vi "Autonomous Independent.vi"() -> ()   [LabVIEW 2016]
doc: "This VI is called when autonomous begins, and will automatically be terminated when autonomous ends. You can carry out timed or sensor driven robot movement independently without needing to return to the caller."
uses:
  <vilib>/Rock Robotics/WPI/ThirdParty/CanMotor/TalonSRX/WPI_CANTalonSRX_APIFeedbackSelect.ctl
  <vilib>/Rock Robotics/WPI/ThirdParty/CanMotor/TalonSRX/WPI_CANTalonSRX_Params.ctl
  <vilib>/Rock Robotics/WPI/ThirdParty/CanMotor/TalonSRX/WPI_CANTalonSRX_APIControlMode.ctl
  <vilib>/Rock Robotics/WPI/Utilities/WPI_GetSetVariantRefNum.vi
  <vilib>/Rock Robotics/Network Tables/NT Read String.vi
  <vilib>/Rock Robotics/Network Tables/NT Write Numeric Array.vi
  Robot Global Data.vi
  <vilib>/Rock Robotics/WPI/RobotDrive/WPI_RobotDriveArcadeDrive_Standard(NoSaturation).vi
panel:
  out "TEST 3":dbl
  out "Encoder Position 7":dbl
  out "Encoder Position 6":dbl
  out "RIGHT SIDE":dbl
  out "Encoder Position 4":dbl
  out "Encoder Position 3":dbl
  out "Encoder Position":dbl
  out "Encoder Position 2":dbl
  # "Be sure to right-click and choose Data Operations>>Make Current Value default if you want to save the array values with the VI"
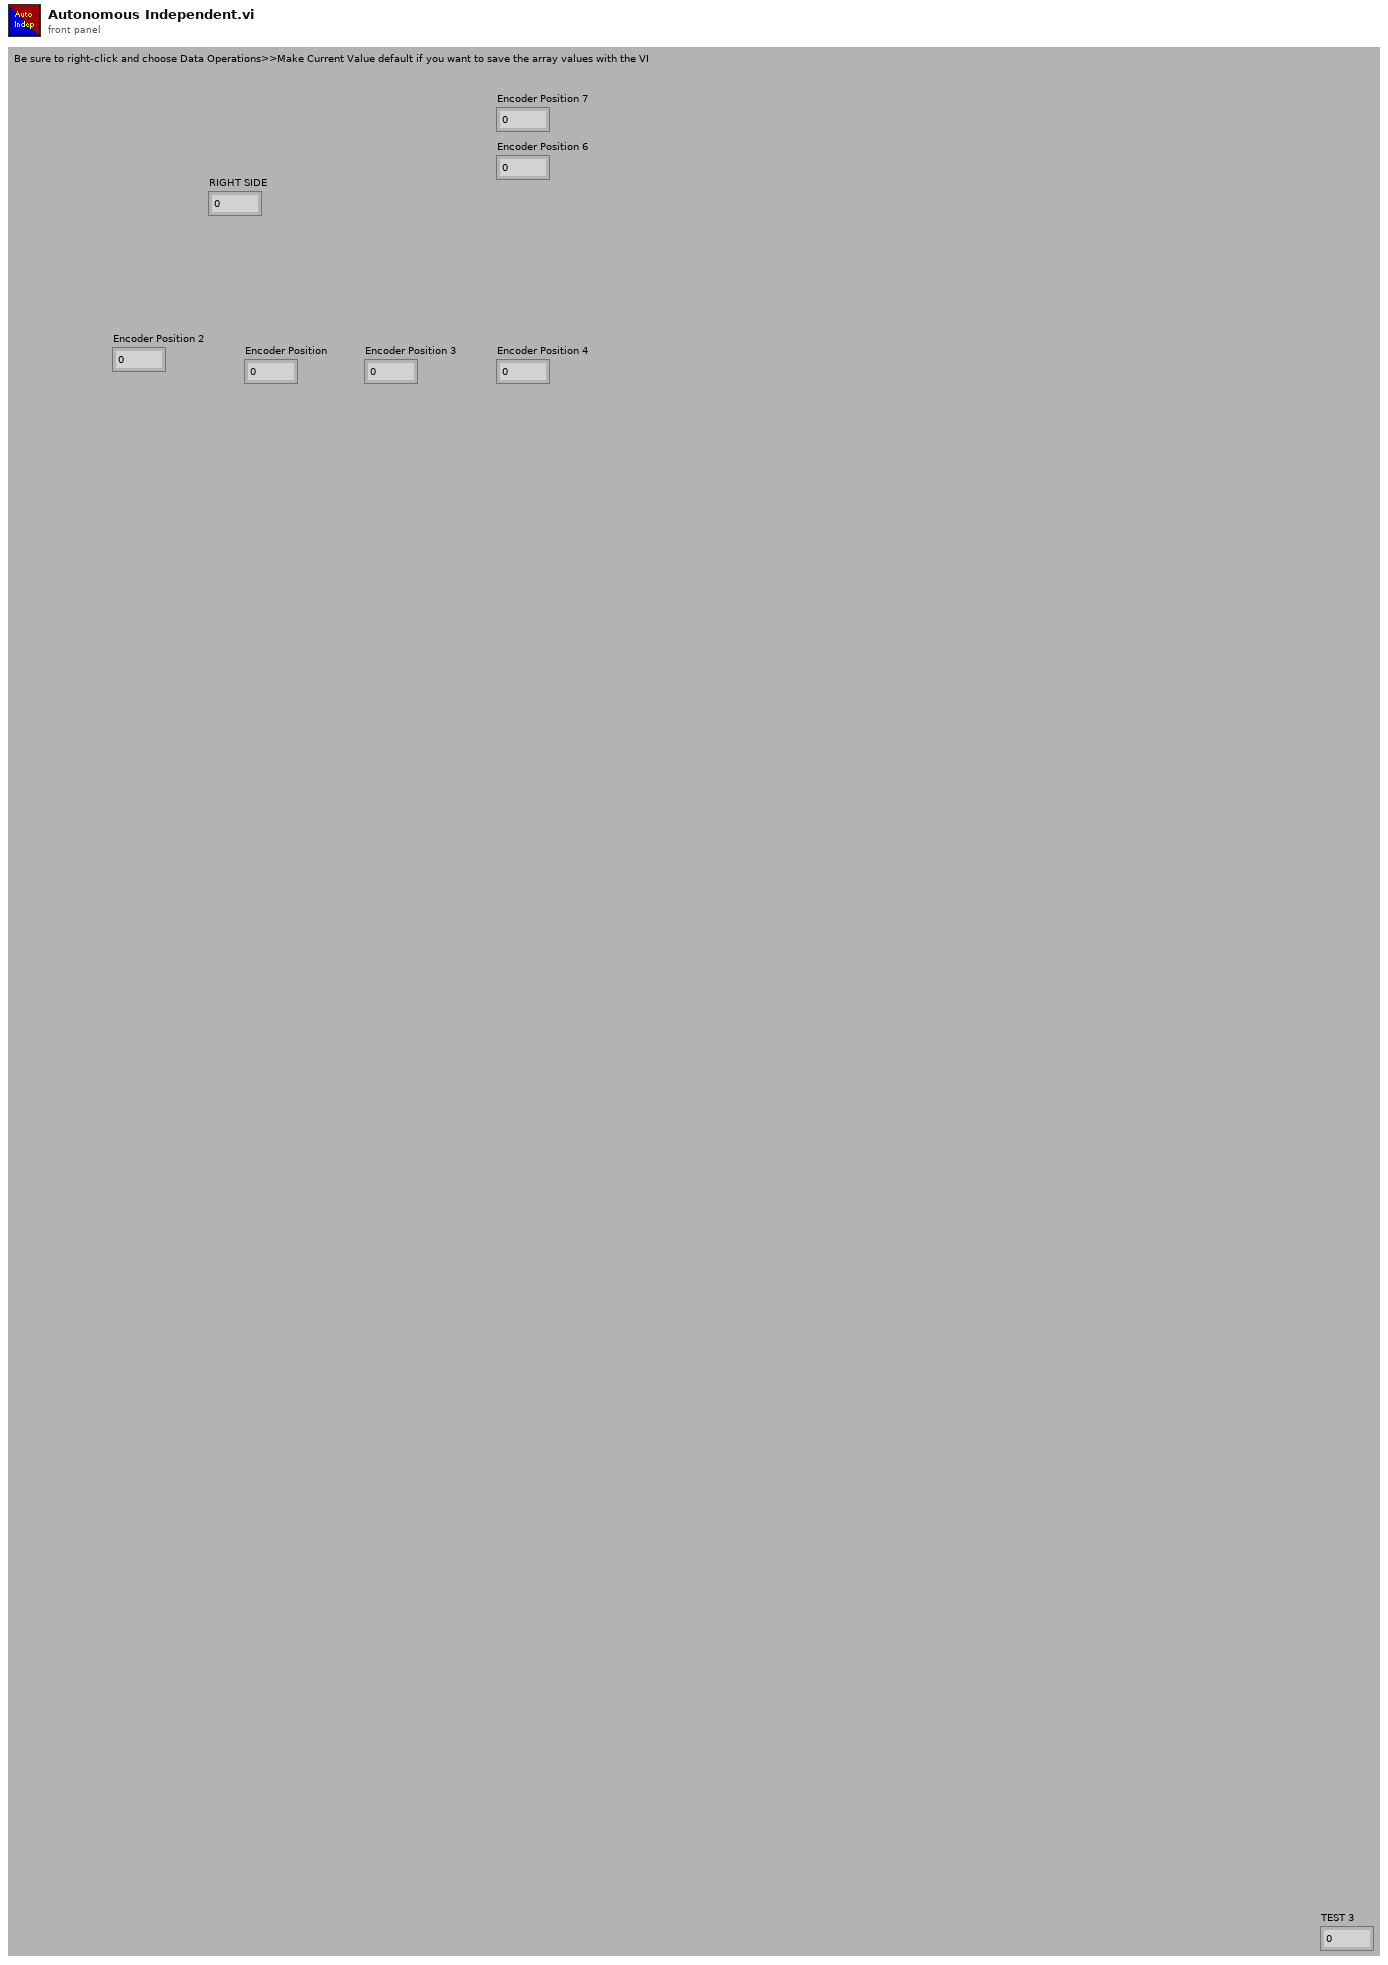
[diagram p1: front panel]
types:
  T1 = typedef "WPI_CANTalonSRX_APIFeedbackSelect.ctl" = enum16{"Digital Quadrature Encoder", "Analog Potentiometer", "Analog Encoder", "Count on Quad-A (Rising-Edge)", "Count on Quad-A (Falling-Edge)", "CTR Magnetic Enc (Absolute)", "CTR Magnetic Enc (Relative)", "Pulse Width"}
  T2 = typedef "WPI_JoystickDevRef.ctl" = cluster{"Device":T3}
  T3 = typedef "WPI_JoystickDeviceEnum.ctl" = enum16{"USB 0", "USB 1", "USB 2", "USB 3", "USB 4", "USB 5"}
  T4 = typedef "WPI_MotorControlDeviceRef.ctl" = cluster{"DeviceStatus":errorcluster, "Type":T5, "PWM":cluster{"PWM Channel":T6, "DeadBand":T7}, "CAN":cluster{"Device Number":u8, "SetOutput VI Ref":variant, "GetOutput VI Ref":variant, "Enable VI Ref":variant, "Disable VI Ref":variant, "Data":variant}, "Invert":bool}
  T5 = typedef "WPI_MotorControlType.ctl" = enum16{"PWM", "CAN"}
  T6 = typedef "FPGA_DIOPWMChannel.ctl" = enum8{"PWM 0", "PWM 1", "PWM 2", "PWM 3", "PWM 4", "PWM 5", "PWM 6", "PWM 7", "PWM 8", "PWM 9", "PWM MXP 0", "PWM MXP 1", "PWM MXP 2", "PWM MXP 3", "PWM MXP 4", "PWM MXP 5", "PWM MXP 6", "PWM MXP 7", "PWM MXP 8", "PWM MXP 9", "Invalid"}
  T7 = typedef "WPI_PWMDeadband.ctl" = cluster{"Name":string, "maxPositivePwm":i32, "minPositivePwm":i32, "centerPwm":i32, "maxNegativePwm":i32, "minNegativePwm":i32, "angularRange":u16}
  T8 = typedef "WPI_CANTalonSRX_GlobalStatus.ctl" = cluster{"Applied Throttle":dbl, "Module Enabled":bool, "CAN Error":errorcluster, "Closed Loop Error":dbl, "Forward Limit Switch Closed":bool, "Reverse Limit Switch Closed":bool, "Sensor Position":dbl, "Sensor Velocity":dbl, "Current":dbl, "Sticky Fault - Over Temp":bool, "Sticky Fault - Under Voltage":bool, "Sticky Fault - Forward Limit":bool, "Sticky Fault - Reverse Limit":bool, "Sticky Fault - Forward Soft Limit":bool, "Sticky Fault - Reverse Soft Limit":bool, "Brake is Enabled":bool, "Encoder Position":dbl, "Encoder Velocity":dbl, "Encoder Index Count":dbl, "Encoder A Pin State":bool, "Encoder B Pin State":bool, "Encoder Index Pin State":bool, "Analog In":dbl, "Analog In Velocity":dbl, "Temperature (C)":dbl, "Battery Voltage":dbl, "Control 5 Is Supported":bool, "Current Profile Slot Select":dbl, "Pos Div 8":bool, "Vel Div 4":bool, "Pulse Width Position":i32, "Pulse Width Velocity":i32, "Pulse Width Rise To Rise (us)":i32, "Pulse Width Rise To Fall (us)":i32, "Mot Prof Active Is Under Run":bool, "Mot Prof Active Has Under Run":bool, "Mot Prof Active Is Last":bool, "Mot Prof Active Velocity Only":bool, "Mot Prof Active Is Valid":bool, "Mot Prof Buffer Is Full":bool, "Mot Prof Active Profile Slot Select":i32, "Mot Prof NextID":i32, "Mot Prof Count":i32, "Mot Prof Active Velocity":dbl, "Mot Prof Active Position":dbl, "Mot Prof Output Enable":i32, "UsageFrame":u32}
  T9 = typedef "WPI_RobotDriveDevRef.ctl" = cluster{"DevStatus":errorcluster, "Motors[]":T4[], "Square Inputs":bool, "Max Output":dbl}
  T10 = typedef "WPI_CANTalonSRX_APIControlMode.ctl" = enum8{"Percent VBus", "Speed", "Position", "Slave", "Unchanged / Invalid", "Voltage Compensation", "Current", "Motion Profile", "Motion Magic"}
  T11 = typedef "WPI_CANTalonSRX_Params.ctl" = u8
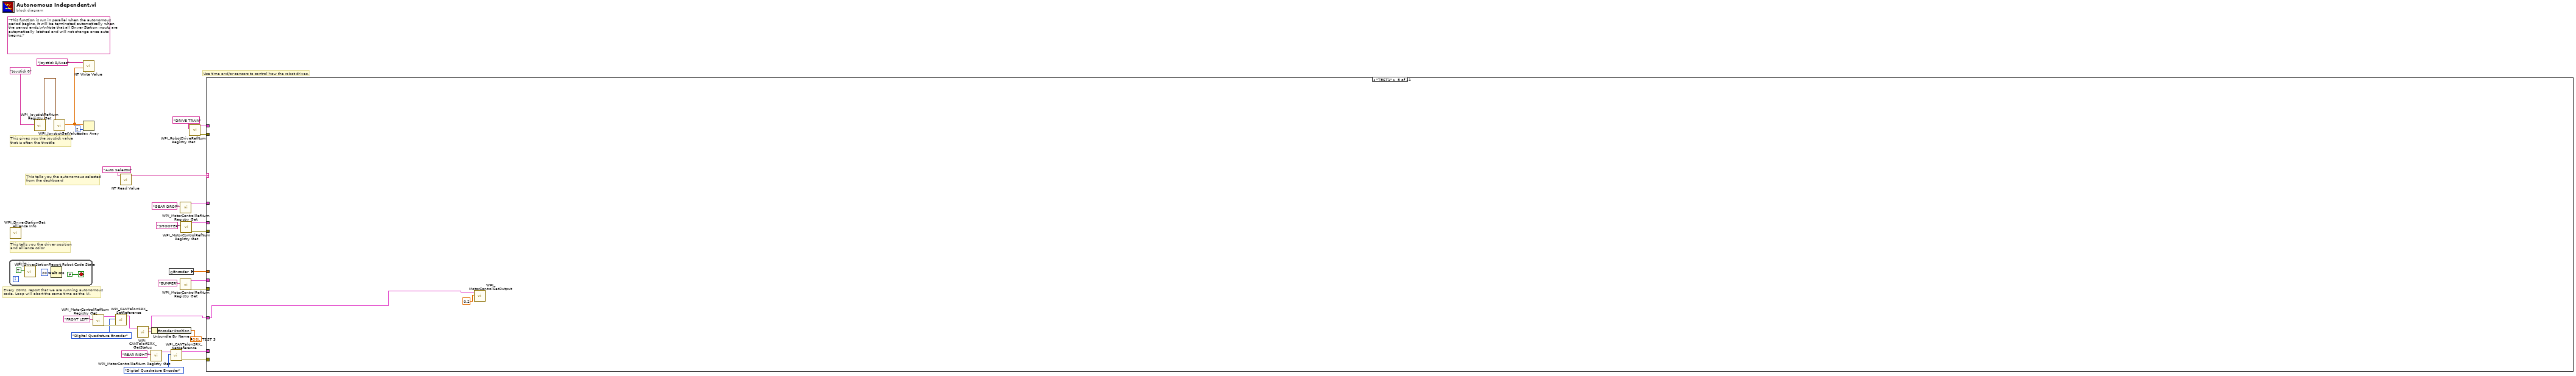
[diagram p0: block diagram]
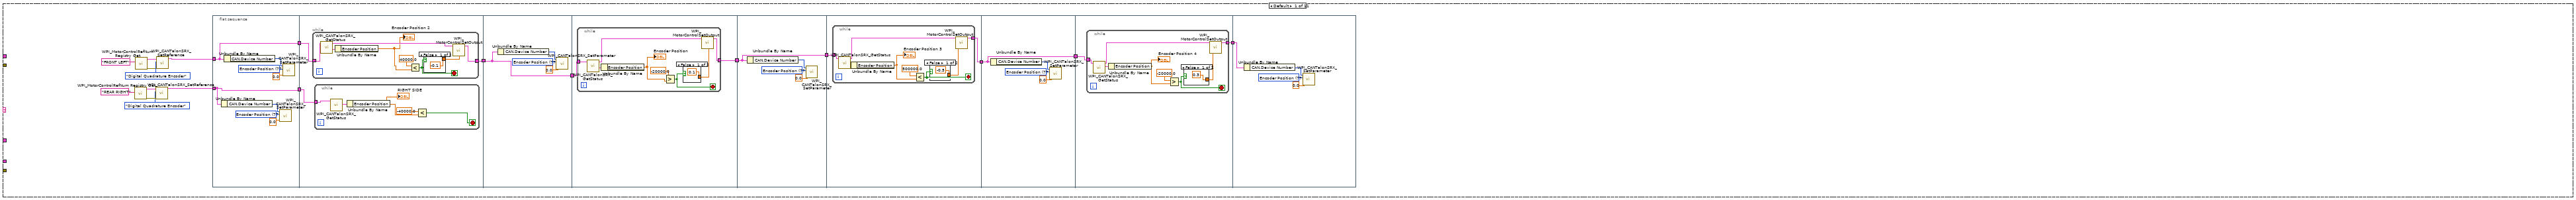
[diagram p2: hidden frame]
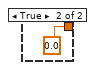
[diagram p3: hidden frame]
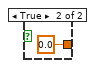
[diagram p4: hidden frame]
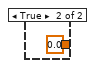
[diagram p5: hidden frame]
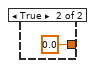
[diagram p6: hidden frame]
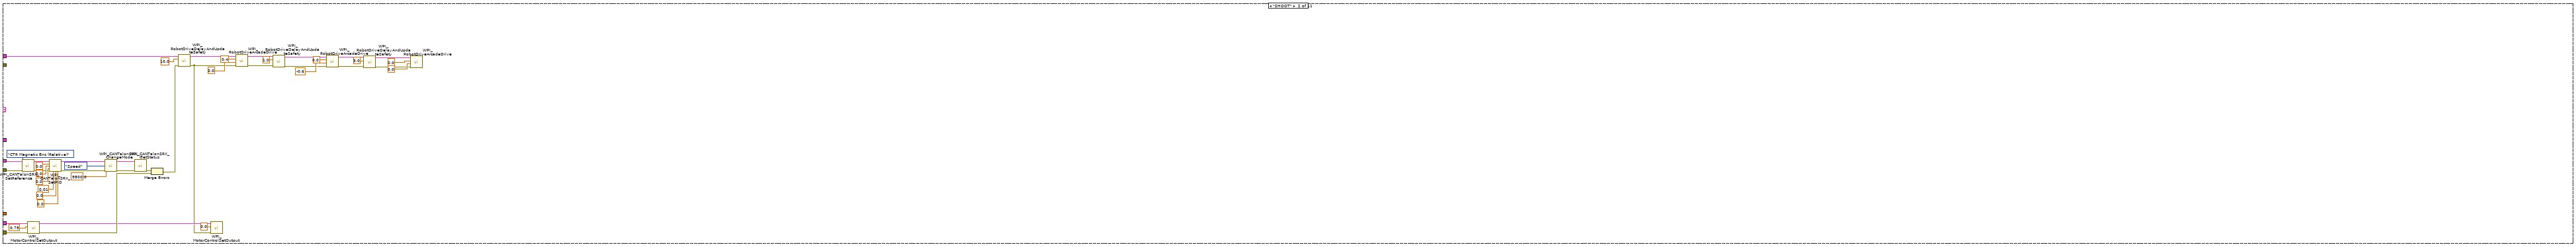
[diagram p7: hidden frame]
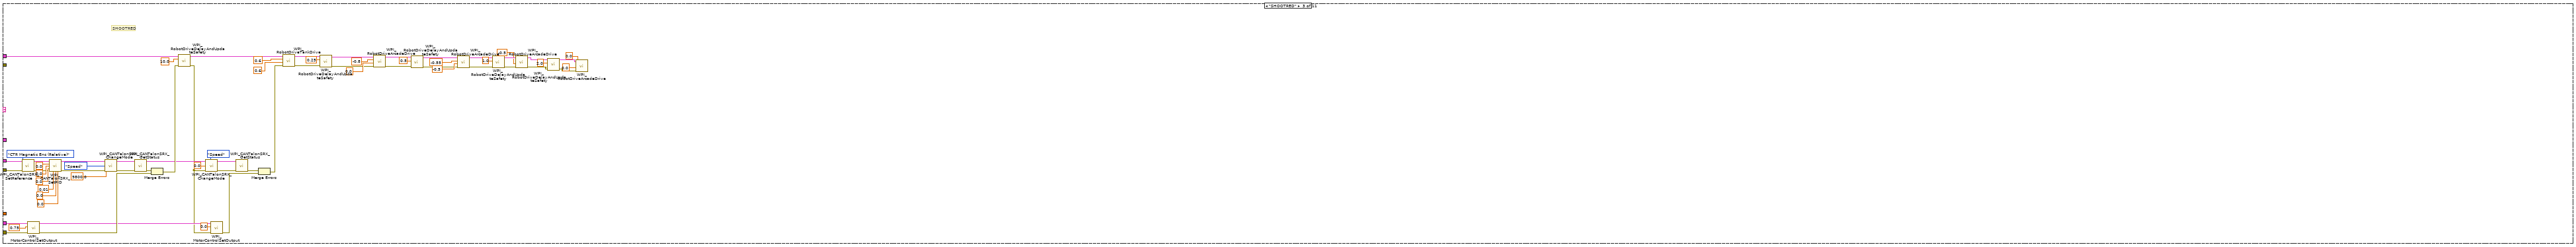
[diagram p8: hidden frame]
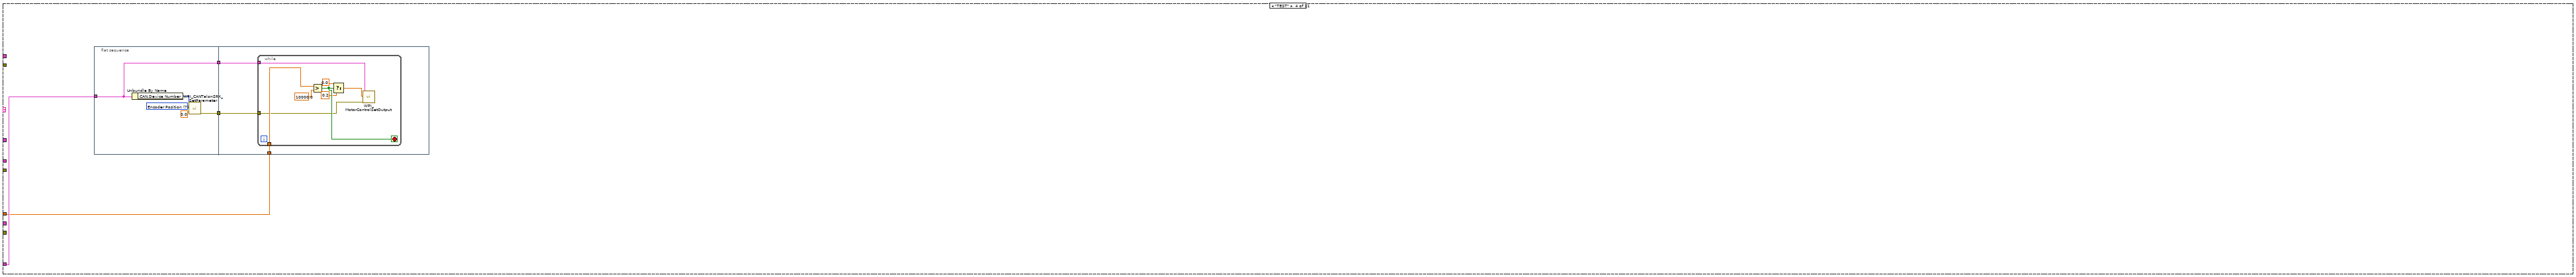
[diagram p9: hidden frame]
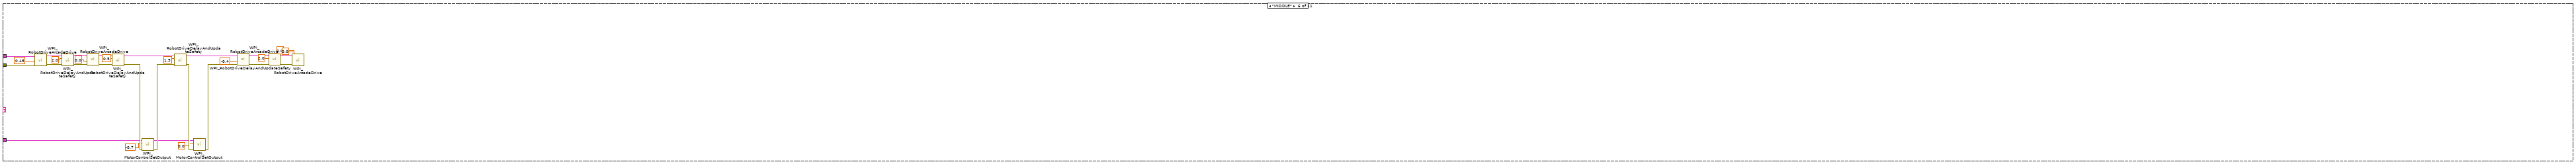
[diagram p10: hidden frame]
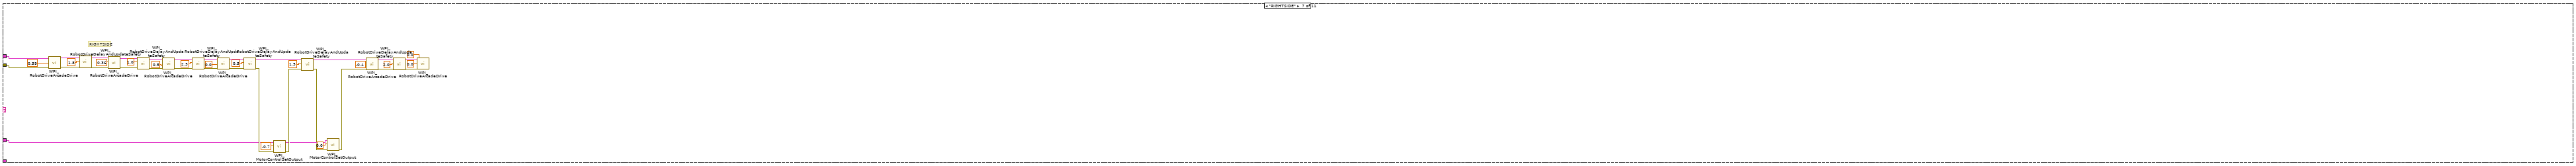
[diagram p11: hidden frame]
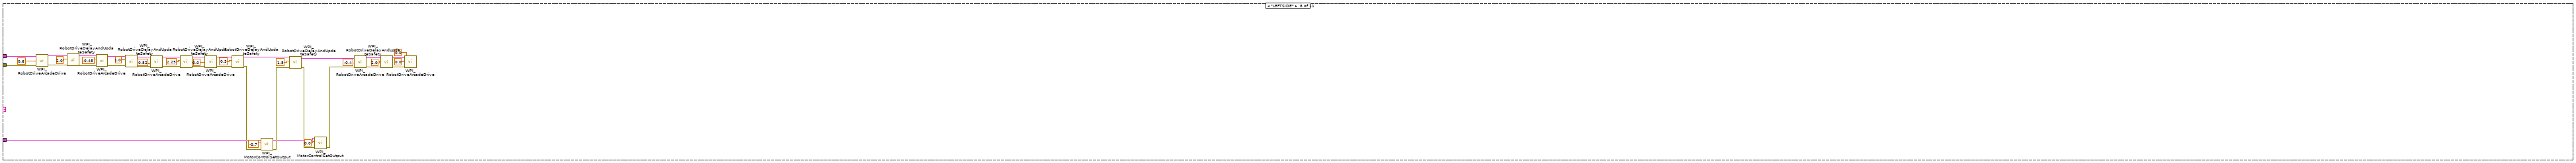
[diagram p12: hidden frame]
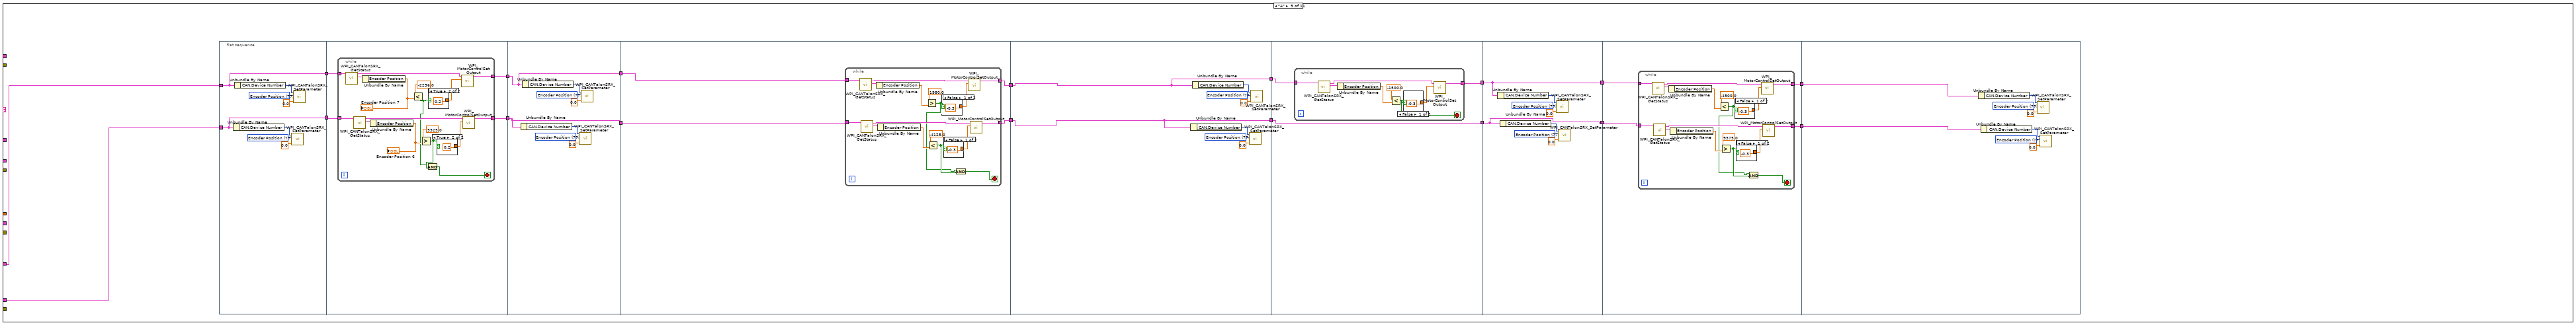
[diagram p13: hidden frame]
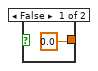
[diagram p14: hidden frame]
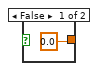
[diagram p15: hidden frame]
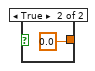
[diagram p16: hidden frame]
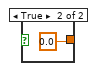
[diagram p17: hidden frame]
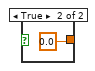
[diagram p18: hidden frame]
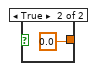
[diagram p19: hidden frame]
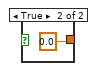
[diagram p20: hidden frame]
diagram:
  (unwired) "This function is run in parallel when the autonomous period begins. It will be terminated automatically when the period ends.\n\nNote that all Driver Station inputs are automatically latched and will not change once auto begins."
  # "Use time and/or sensors to control how the robot drives."
  # "This tells you the autonomous selected\nfrom the dashboard"
  # "Every 20ms, report that we are running autonomous\ncode. Loop will abort the same time as the VI."
  # "This gives you the joystick value\nthat is often the throttle"
  # "This tells you the driver position\nand alliance color"
  n1 = while {
    stop <- FALSE stop-if-true
    n2 = call <vilib>:"WPI_DriverStationReport Robot Code State.vi"("Autonomous"=TRUE) -> ()  [unwired: 10 in, 1 out]
    n3 = Wait (ms)(milliseconds to wait=u32 20) -> ()  [unwired: 1 out]
  }
  n4 = call <vilib>:"WPI_DriverStationGet Alliance Info.vi"() -> ()  [unwired: 12 out]
  n5 = call <vilib>:"WPI_JoystickRefNum Registry Get.vi"("refnum name"="Joystick 0") -> ("JoystickDevRef"=w31:T2)  [unwired: 1 in, 9 out]
  n6 = call <vilib>:"WPI_JoystickGetValues.vi"("JoystickDevRef"=w31) -> ("Axes"=w27:dbl[])  [unwired: 6 in, 4 out]
  n7 = call-poly <vilib>:"NT Write Value.vi"("Numeric Array"=w27, "Name"="Joystick 0/Axes") -> ()  [unwired: 9 in, 1 out]
  n8 = Index Array(array=w27, index=2) -> ()  [unwired: 1 out]
  n9 = call <vilib>:"WPI_MotorControlRefNum Registry Get.vi"("refnum name"="FRONT LEFT") -> ("error out"=w6:errorcluster, "MotorControlDevRef"=w7:T4)  [unwired: 9 in]
  n10 = call <vilib>:"WPI_CANTalonSRX_SetReference.vi"("error in (no error)"=w6, "Feedback Reference"=WPI_CANTalonSRX_APIFeedbackSelect."Digital Quadrature Encoder", "CAN Talon SRX Ref"=w7) -> ("CAN Talon SRX Ref"=w2:T4)  [unwired: 7 in, 1 out]
  n11 = call-poly <vilib>:"NT Read Value.vi"("Name"="Auto Selector") -> ("String"=w28:string)  [unwired: 9 in, 1 out]
  n12 = call <vilib>:"WPI_CANTalonSRX_GetStatus.vi"("CAN Talon SRX Ref"=w2) -> ("Talon SRX Status"=w4:T8, "CAN Talon SRX Ref"=w1:T4)  [unwired: 8 in, 1 out]
  n13 = call <vilib>:"WPI_MotorControlRefNum Registry Get.vi"("refnum name"="REAR RIGHT") -> ("MotorControlDevRef"=w23:T4)  [unwired: 9 in, 1 out]
  n14 = Unbundle By Name(w4) -> ("Encoder Position"=→"TEST 3":dbl)
  n15 = global read "Robot Global Data.vi" "Encoder"() -> (w8:dbl)
  n16 = call <vilib>:"WPI_CANTalonSRX_SetReference.vi"("Feedback Reference"=WPI_CANTalonSRX_APIFeedbackSelect."Digital Quadrature Encoder", "CAN Talon SRX Ref"=w23) -> ("error out"=w20:errorcluster, "CAN Talon SRX Ref"=w21:T4)  [unwired: 8 in]
  n17 = call <vilib>:"WPI_MotorControlRefNum Registry Get.vi"("refnum name"="GEAR DROP") -> ("MotorControlDevRef"=w15:T4)  [unwired: 9 in, 1 out]
  n18 = call <vilib>:"WPI_MotorControlRefNum Registry Get.vi"("refnum name"="BUMPER") -> ("error out"=w10:errorcluster, "MotorControlDevRef"=w11:T4)  [unwired: 9 in]
  n19 = call <vilib>:"WPI_MotorControlRefNum Registry Get.vi"("refnum name"="SHOOTER") -> ("error out"=w12:errorcluster, "MotorControlDevRef"=w13:T4)  [unwired: 9 in]
  n20 = call <vilib>:"WPI_RobotDriveRefNum Registry Get.vi"("refnum name"="DRIVE TRAIN") -> ("error out"=w17:errorcluster, "RobotDriveDevRef"=w18:T9)  [unwired: 9 in]
  n21 = case shown="\"TEST1\"" w28 {
    tunnel: w21 -> [_ _ _ _ _ _ _ _ w389 _ _]
    tunnel: w20 -> [_ _ _ _ _ _ _ _ _ _ _]
    tunnel: w18 -> [_ w159 w225 _ _ w296 w299 w382 _ w534 w559]
    tunnel: w17 -> [_ _ _ _ _ w295 w298 w381 _ w533 w558]
    tunnel: w15 -> [_ _ _ _ _ w283 w297 w358 _ _ w539]
    tunnel: w13 -> [_ w165 w231 _ _ _ _ _ _ _ _]
    tunnel: w12 -> [_ w164 w230 _ _ _ _ _ _ _ _]
    tunnel: w11 -> [_ w150 w218 _ _ _ _ _ _ _ _]
    tunnel: w10 -> [_ w149 w217 _ _ _ _ _ _ _ _]
    tunnel: w1 -> [_ _ _ w247 w264 _ _ _ w384 _ _]
    tunnel: w8 -> [_ _ _ w246 _ _ _ _ _ _ _]
    frame Default {
      n22 = call <vilib>:"WPI_MotorControlRefNum Registry Get.vi"("refnum name"="REAR RIGHT") -> ("error out"=w40:errorcluster, "MotorControlDevRef"=w39:T4)  [unwired: 9 in]
      n23 = call <vilib>:"WPI_MotorControlRefNum Registry Get.vi"("refnum name"="FRONT LEFT") -> ("error out"=w52:errorcluster, "MotorControlDevRef"=w53:T4)  [unwired: 9 in]
      n24 = call <vilib>:"WPI_CANTalonSRX_SetReference.vi"("error in (no error)"=w40, "Feedback Reference"=WPI_CANTalonSRX_APIFeedbackSelect."Digital Quadrature Encoder", "CAN Talon SRX Ref"=w39) -> ("CAN Talon SRX Ref"=w37:T4)  [unwired: 7 in, 1 out]
      n25 = call <vilib>:"WPI_CANTalonSRX_SetReference.vi"("error in (no error)"=w52, "Feedback Reference"=WPI_CANTalonSRX_APIFeedbackSelect."Digital Quadrature Encoder", "CAN Talon SRX Ref"=w53) -> ("CAN Talon SRX Ref"=w48:T4)  [unwired: 7 in, 1 out]
      n26 = flat-sequence {
        tunnel: w48 -> [w59]
        tunnel: [w59] -> w47
        tunnel: w37 -> [w55]
        tunnel: [w55] -> w36
        tunnel: [w64] -> w50
        tunnel: w47 -> [w65]
        tunnel: w36 -> [w63]
        tunnel: w50 -> [w81]
        tunnel: [w81] -> w49
        tunnel: w49 -> [w86]
        tunnel: [w85] -> w46
        tunnel: w46 -> [w97]
        tunnel: [w97] -> w45
        tunnel: w45 -> [w102]
        tunnel: [w101] -> w44
        tunnel: w44 -> [w113]
        tunnel: [w113] -> w43
        tunnel: w43 -> [w118]
        tunnel: [w117] -> w42
        tunnel: w42 -> [w129]
        frame #0 {
          w57 = T11 77 items=["Slot 0 - P"=1, "Slot 0 - I"=2, "Slot 0 - D"=3, "Slot 0 - F"=4, "Slot 0 - I Zone"=5, "Slot 0 - Ramp Rate"=6, "Slot 1 - P"=11, "Slot 1 - I"=12, "Slot 1 - D"=13, "Slot 1 - F"=14, "Slot 1 - I Zone"=15, "Slot 1 - Ramp Rate"=16, "Soft Limit - Forward"=21, "Soft Limit - Reverse"=22, "Soft Limit - Forward Enable"=23, "Soft Limit - Reverse Enable"=24, "On Boot - Brake Mode"=31, "On Boot - Limit Normally Closed - Forward"=32, "On Boot - Limit Normally Closed - Reverse"=33, "On Boot - Limit Disabled - Forward"=34, "On Boot - Limit Disabled - Reverse"=35, "Fault - Over Temp"=41, "Fault - Under Voltage"=42, "Fault - Forward Limit"=43, "Fault - Reverse Limit"=44, "Fault - Hardware Failure"=45, "Fault - Forward Soft Limit"=46, "Fault - Reverse Soft Limit"=47, "Sticky Fault - Over Temp"=48, "Sticky Fault - Under Voltage"=49, "Sticky Fault - Forward Limit"=50, "Sticky Fault - Reverse Limit"=51, "Sticky Fault - Forward Soft Limit"=52, "Sticky Fault - Reverse Soft Limit"=53, "Applied Throttle"=61, "Closed-Loop Error"=62, "Select Feedback Device"=63, "Reverse Closed-Loop Output"=64, "Mode Select"=65, "Profile Slot Select"=66, "Ramp Throttle"=67, "Reverse Feedback Sensor"=68, "Limit Switch Enabled"=69, "Limit Switch Closed - Forward"=70, "Limit Switch Closed - Reverse"=71, "Sensor Position"=73, "Sensor Velocity"=74, "Current"=75, "Brake is Enabled"=76, "Encoder Position"=77, "Encoder Velocity"=78, "Encoder Index Rise Events"=79, "Encoder A Pin State"=80, "Encoder B Pin State"=81, "Encoder Index Pin State"=82, "Analog In with Overflow"=83, "Analog In Velocity"=84, "Temperature"=85, "Battery Voltage"=86, "Reset Count"=87, "Reset Flags"=88, "Firmware Version"=89, "Settings Changed"=90, "Quad Filter Enable"=91, "Ignore Disable Broadcast"=92, "I Accumulator"=93, "Status 1 Frame Rate Ms"=94, "Status 2 Frame Rate Ms"=95, "Status 3 Frame Rate Ms"=96, "Status 4 Frame Rate Ms"=97, "Status 6 Frame Rate Ms"=98, "Status 7 Frame Rate Ms"=99, "Enable Index Pin Clear Position"=100, "Peak Positive Output"=104, "Nominal Positive Output"=105, "Peak Negative Output"=106, "Nominal Negative Output"=107, "Quad Index Pin Polarity"=108, "Status 8 Frame Rate Ms"=109, "Allow Position Overflow"=110, "Slot 0 - Allowable Closed-Loop Error"=111, "Number Potentiometer Turns"=112, "Encoder Codes Per Rev"=113, "Pulse Width Decoded Position"=114, "Analog Position"=115, "Voltage Compensation Rate (V/s)"=116, "Slot 1 - Allowable Closed-Loop Error"=117, "Motion Profile Has Underrun Err"=119, "Reserved 120"=120, "Legacy Control Mode"=121, "Motion Magic Acceleration"=122, "Motion Magic Cruise Velocity"=123, "Status 10 Frame Rate"=124, "Current Limit Threshold"=125, "CustomParam0"=137, "CustomParam1"=138, "PersStorageSaving"=139, "ClearPositionOnLimitF"=144, "ClearPositionOnLimitR"=145, "NominalBatteryVoltage"=146, "SampleVelocityPeriod"=147, "SampleVelocityWindow"=148] ("Parameter")
          w61 = T11 77 items=["Slot 0 - P"=1, "Slot 0 - I"=2, "Slot 0 - D"=3, "Slot 0 - F"=4, "Slot 0 - I Zone"=5, "Slot 0 - Ramp Rate"=6, "Slot 1 - P"=11, "Slot 1 - I"=12, "Slot 1 - D"=13, "Slot 1 - F"=14, "Slot 1 - I Zone"=15, "Slot 1 - Ramp Rate"=16, "Soft Limit - Forward"=21, "Soft Limit - Reverse"=22, "Soft Limit - Forward Enable"=23, "Soft Limit - Reverse Enable"=24, "On Boot - Brake Mode"=31, "On Boot - Limit Normally Closed - Forward"=32, "On Boot - Limit Normally Closed - Reverse"=33, "On Boot - Limit Disabled - Forward"=34, "On Boot - Limit Disabled - Reverse"=35, "Fault - Over Temp"=41, "Fault - Under Voltage"=42, "Fault - Forward Limit"=43, "Fault - Reverse Limit"=44, "Fault - Hardware Failure"=45, "Fault - Forward Soft Limit"=46, "Fault - Reverse Soft Limit"=47, "Sticky Fault - Over Temp"=48, "Sticky Fault - Under Voltage"=49, "Sticky Fault - Forward Limit"=50, "Sticky Fault - Reverse Limit"=51, "Sticky Fault - Forward Soft Limit"=52, "Sticky Fault - Reverse Soft Limit"=53, "Applied Throttle"=61, "Closed-Loop Error"=62, "Select Feedback Device"=63, "Reverse Closed-Loop Output"=64, "Mode Select"=65, "Profile Slot Select"=66, "Ramp Throttle"=67, "Reverse Feedback Sensor"=68, "Limit Switch Enabled"=69, "Limit Switch Closed - Forward"=70, "Limit Switch Closed - Reverse"=71, "Sensor Position"=73, "Sensor Velocity"=74, "Current"=75, "Brake is Enabled"=76, "Encoder Position"=77, "Encoder Velocity"=78, "Encoder Index Rise Events"=79, "Encoder A Pin State"=80, "Encoder B Pin State"=81, "Encoder Index Pin State"=82, "Analog In with Overflow"=83, "Analog In Velocity"=84, "Temperature"=85, "Battery Voltage"=86, "Reset Count"=87, "Reset Flags"=88, "Firmware Version"=89, "Settings Changed"=90, "Quad Filter Enable"=91, "Ignore Disable Broadcast"=92, "I Accumulator"=93, "Status 1 Frame Rate Ms"=94, "Status 2 Frame Rate Ms"=95, "Status 3 Frame Rate Ms"=96, "Status 4 Frame Rate Ms"=97, "Status 6 Frame Rate Ms"=98, "Status 7 Frame Rate Ms"=99, "Enable Index Pin Clear Position"=100, "Peak Positive Output"=104, "Nominal Positive Output"=105, "Peak Negative Output"=106, "Nominal Negative Output"=107, "Quad Index Pin Polarity"=108, "Status 8 Frame Rate Ms"=109, "Allow Position Overflow"=110, "Slot 0 - Allowable Closed-Loop Error"=111, "Number Potentiometer Turns"=112, "Encoder Codes Per Rev"=113, "Pulse Width Decoded Position"=114, "Analog Position"=115, "Voltage Compensation Rate (V/s)"=116, "Slot 1 - Allowable Closed-Loop Error"=117, "Motion Profile Has Underrun Err"=119, "Reserved 120"=120, "Legacy Control Mode"=121, "Motion Magic Acceleration"=122, "Motion Magic Cruise Velocity"=123, "Status 10 Frame Rate"=124, "Current Limit Threshold"=125, "CustomParam0"=137, "CustomParam1"=138, "PersStorageSaving"=139, "ClearPositionOnLimitF"=144, "ClearPositionOnLimitR"=145, "NominalBatteryVoltage"=146, "SampleVelocityPeriod"=147, "SampleVelocityWindow"=148] ("Parameter")
          n27 = Unbundle By Name(w55) -> ("CAN.Device Number"=w56:u8)
          n28 = Unbundle By Name(w59) -> ("CAN.Device Number"=w62:u8)
          n29 = call <vilib>:"WPI_CANTalonSRX_SetParameter.vi"("Value"=0.0, "Parameter"=w57, "Device ID (0)"=w56) -> ()  [unwired: 7 in, 2 out]
          n30 = call <vilib>:"WPI_CANTalonSRX_SetParameter.vi"("Value"=0.0, "Parameter"=w61, "Device ID (0)"=w62) -> ()  [unwired: 7 in, 2 out]
        }
        frame #1 {
          n31 = while {
            tunnel: w65 -> [w72]
            tunnel: [w71] -> w64
            stop <- w75 stop-if-true
            n32 = call <vilib>:"WPI_CANTalonSRX_GetStatus.vi"("CAN Talon SRX Ref"=w72) -> ("Talon SRX Status"=w78:T8, "CAN Talon SRX Ref"=w77:T4)  [unwired: 8 in, 1 out]
            n33 = Unbundle By Name(w78) -> ("Encoder Position"=w74:dbl)
            "Encoder Position 2" <- w74
            n34 = Less?(x=40000.0, y=w74) -> (x < y?=w75:bool)
            n35 = case shown="False" w75 {
              tunnel: [-0.1 ("x") 0.0 ("x")] -> w76
              frame False {
              }
              frame True {
              }
            }
            n36 = call <vilib>:"WPI_MotorControlSetOutput.vi"("Output"=w76, "MotorControlDevRef"=w77) -> ("MotorControlDevRef"=w71:T4)  [unwired: 7 in, 2 out]
          }
          n37 = while {
            tunnel: w63 -> [w70]
            stop <- w67 stop-if-true
            n38 = call <vilib>:"WPI_CANTalonSRX_GetStatus.vi"("CAN Talon SRX Ref"=w70) -> ("Talon SRX Status"=w66:T8)  [unwired: 8 in, 2 out]
            n39 = Unbundle By Name(w66) -> ("Encoder Position"=w69:dbl)
            "RIGHT SIDE" <- w69
            n40 = Less?(x=-40000.0, y=w69) -> (x < y?=w67:bool)
          }
        }
        frame #2 {
          w83 = T11 77 items=["Slot 0 - P"=1, "Slot 0 - I"=2, "Slot 0 - D"=3, "Slot 0 - F"=4, "Slot 0 - I Zone"=5, "Slot 0 - Ramp Rate"=6, "Slot 1 - P"=11, "Slot 1 - I"=12, "Slot 1 - D"=13, "Slot 1 - F"=14, "Slot 1 - I Zone"=15, "Slot 1 - Ramp Rate"=16, "Soft Limit - Forward"=21, "Soft Limit - Reverse"=22, "Soft Limit - Forward Enable"=23, "Soft Limit - Reverse Enable"=24, "On Boot - Brake Mode"=31, "On Boot - Limit Normally Closed - Forward"=32, "On Boot - Limit Normally Closed - Reverse"=33, "On Boot - Limit Disabled - Forward"=34, "On Boot - Limit Disabled - Reverse"=35, "Fault - Over Temp"=41, "Fault - Under Voltage"=42, "Fault - Forward Limit"=43, "Fault - Reverse Limit"=44, "Fault - Hardware Failure"=45, "Fault - Forward Soft Limit"=46, "Fault - Reverse Soft Limit"=47, "Sticky Fault - Over Temp"=48, "Sticky Fault - Under Voltage"=49, "Sticky Fault - Forward Limit"=50, "Sticky Fault - Reverse Limit"=51, "Sticky Fault - Forward Soft Limit"=52, "Sticky Fault - Reverse Soft Limit"=53, "Applied Throttle"=61, "Closed-Loop Error"=62, "Select Feedback Device"=63, "Reverse Closed-Loop Output"=64, "Mode Select"=65, "Profile Slot Select"=66, "Ramp Throttle"=67, "Reverse Feedback Sensor"=68, "Limit Switch Enabled"=69, "Limit Switch Closed - Forward"=70, "Limit Switch Closed - Reverse"=71, "Sensor Position"=73, "Sensor Velocity"=74, "Current"=75, "Brake is Enabled"=76, "Encoder Position"=77, "Encoder Velocity"=78, "Encoder Index Rise Events"=79, "Encoder A Pin State"=80, "Encoder B Pin State"=81, "Encoder Index Pin State"=82, "Analog In with Overflow"=83, "Analog In Velocity"=84, "Temperature"=85, "Battery Voltage"=86, "Reset Count"=87, "Reset Flags"=88, "Firmware Version"=89, "Settings Changed"=90, "Quad Filter Enable"=91, "Ignore Disable Broadcast"=92, "I Accumulator"=93, "Status 1 Frame Rate Ms"=94, "Status 2 Frame Rate Ms"=95, "Status 3 Frame Rate Ms"=96, "Status 4 Frame Rate Ms"=97, "Status 6 Frame Rate Ms"=98, "Status 7 Frame Rate Ms"=99, "Enable Index Pin Clear Position"=100, "Peak Positive Output"=104, "Nominal Positive Output"=105, "Peak Negative Output"=106, "Nominal Negative Output"=107, "Quad Index Pin Polarity"=108, "Status 8 Frame Rate Ms"=109, "Allow Position Overflow"=110, "Slot 0 - Allowable Closed-Loop Error"=111, "Number Potentiometer Turns"=112, "Encoder Codes Per Rev"=113, "Pulse Width Decoded Position"=114, "Analog Position"=115, "Voltage Compensation Rate (V/s)"=116, "Slot 1 - Allowable Closed-Loop Error"=117, "Motion Profile Has Underrun Err"=119, "Reserved 120"=120, "Legacy Control Mode"=121, "Motion Magic Acceleration"=122, "Motion Magic Cruise Velocity"=123, "Status 10 Frame Rate"=124, "Current Limit Threshold"=125, "CustomParam0"=137, "CustomParam1"=138, "PersStorageSaving"=139, "ClearPositionOnLimitF"=144, "ClearPositionOnLimitR"=145, "NominalBatteryVoltage"=146, "SampleVelocityPeriod"=147, "SampleVelocityWindow"=148] ("Parameter")
          n41 = Unbundle By Name(w81) -> ("CAN.Device Number"=w84:u8)
          n42 = call <vilib>:"WPI_CANTalonSRX_SetParameter.vi"("Value"=0.0, "Parameter"=w83, "Device ID (0)"=w84) -> ()  [unwired: 7 in, 2 out]
        }
        frame #3 {
          n43 = while {
            tunnel: w86 -> [w88]
            tunnel: [w87] -> w85
            stop <- w91 stop-if-true
            n44 = call <vilib>:"WPI_CANTalonSRX_GetStatus.vi"("CAN Talon SRX Ref"=w88) -> ("Talon SRX Status"=w94:T8, "CAN Talon SRX Ref"=w93:T4)  [unwired: 8 in, 1 out]
            n45 = Unbundle By Name(w94) -> ("Encoder Position"=w90:dbl)
            "Encoder Position" <- w90
            n46 = Greater?(x=-20000.0 ("y"), y=w90) -> (0:w91:bool)
            n47 = case shown="False" w91 {
              tunnel: [0.1 ("x") 0.0 ("x")] -> w92
              frame False {
              }
              frame True {
              }
            }
            n48 = call <vilib>:"WPI_MotorControlSetOutput.vi"("Output"=w92, "MotorControlDevRef"=w93) -> ("MotorControlDevRef"=w87:T4)  [unwired: 7 in, 2 out]
          }
        }
        frame #4 {
          w99 = T11 77 items=["Slot 0 - P"=1, "Slot 0 - I"=2, "Slot 0 - D"=3, "Slot 0 - F"=4, "Slot 0 - I Zone"=5, "Slot 0 - Ramp Rate"=6, "Slot 1 - P"=11, "Slot 1 - I"=12, "Slot 1 - D"=13, "Slot 1 - F"=14, "Slot 1 - I Zone"=15, "Slot 1 - Ramp Rate"=16, "Soft Limit - Forward"=21, "Soft Limit - Reverse"=22, "Soft Limit - Forward Enable"=23, "Soft Limit - Reverse Enable"=24, "On Boot - Brake Mode"=31, "On Boot - Limit Normally Closed - Forward"=32, "On Boot - Limit Normally Closed - Reverse"=33, "On Boot - Limit Disabled - Forward"=34, "On Boot - Limit Disabled - Reverse"=35, "Fault - Over Temp"=41, "Fault - Under Voltage"=42, "Fault - Forward Limit"=43, "Fault - Reverse Limit"=44, "Fault - Hardware Failure"=45, "Fault - Forward Soft Limit"=46, "Fault - Reverse Soft Limit"=47, "Sticky Fault - Over Temp"=48, "Sticky Fault - Under Voltage"=49, "Sticky Fault - Forward Limit"=50, "Sticky Fault - Reverse Limit"=51, "Sticky Fault - Forward Soft Limit"=52, "Sticky Fault - Reverse Soft Limit"=53, "Applied Throttle"=61, "Closed-Loop Error"=62, "Select Feedback Device"=63, "Reverse Closed-Loop Output"=64, "Mode Select"=65, "Profile Slot Select"=66, "Ramp Throttle"=67, "Reverse Feedback Sensor"=68, "Limit Switch Enabled"=69, "Limit Switch Closed - Forward"=70, "Limit Switch Closed - Reverse"=71, "Sensor Position"=73, "Sensor Velocity"=74, "Current"=75, "Brake is Enabled"=76, "Encoder Position"=77, "Encoder Velocity"=78, "Encoder Index Rise Events"=79, "Encoder A Pin State"=80, "Encoder B Pin State"=81, "Encoder Index Pin State"=82, "Analog In with Overflow"=83, "Analog In Velocity"=84, "Temperature"=85, "Battery Voltage"=86, "Reset Count"=87, "Reset Flags"=88, "Firmware Version"=89, "Settings Changed"=90, "Quad Filter Enable"=91, "Ignore Disable Broadcast"=92, "I Accumulator"=93, "Status 1 Frame Rate Ms"=94, "Status 2 Frame Rate Ms"=95, "Status 3 Frame Rate Ms"=96, "Status 4 Frame Rate Ms"=97, "Status 6 Frame Rate Ms"=98, "Status 7 Frame Rate Ms"=99, "Enable Index Pin Clear Position"=100, "Peak Positive Output"=104, "Nominal Positive Output"=105, "Peak Negative Output"=106, "Nominal Negative Output"=107, "Quad Index Pin Polarity"=108, "Status 8 Frame Rate Ms"=109, "Allow Position Overflow"=110, "Slot 0 - Allowable Closed-Loop Error"=111, "Number Potentiometer Turns"=112, "Encoder Codes Per Rev"=113, "Pulse Width Decoded Position"=114, "Analog Position"=115, "Voltage Compensation Rate (V/s)"=116, "Slot 1 - Allowable Closed-Loop Error"=117, "Motion Profile Has Underrun Err"=119, "Reserved 120"=120, "Legacy Control Mode"=121, "Motion Magic Acceleration"=122, "Motion Magic Cruise Velocity"=123, "Status 10 Frame Rate"=124, "Current Limit Threshold"=125, "CustomParam0"=137, "CustomParam1"=138, "PersStorageSaving"=139, "ClearPositionOnLimitF"=144, "ClearPositionOnLimitR"=145, "NominalBatteryVoltage"=146, "SampleVelocityPeriod"=147, "SampleVelocityWindow"=148] ("Parameter")
          n49 = Unbundle By Name(w97) -> ("CAN.Device Number"=w100:u8)
          n50 = call <vilib>:"WPI_CANTalonSRX_SetParameter.vi"("Value"=0.0, "Parameter"=w99, "Device ID (0)"=w100) -> ()  [unwired: 7 in, 2 out]
        }
        frame #5 {
          n51 = while {
            tunnel: w102 -> [w104]
            tunnel: [w103] -> w101
            stop <- w107 stop-if-true
            n52 = call <vilib>:"WPI_CANTalonSRX_GetStatus.vi"("CAN Talon SRX Ref"=w104) -> ("Talon SRX Status"=w110:T8, "CAN Talon SRX Ref"=w109:T4)  [unwired: 8 in, 1 out]
            n53 = Unbundle By Name(w110) -> ("Encoder Position"=w106:dbl)
            "Encoder Position 3" <- w106
            n54 = Less?(x=500000.0, y=w106) -> (x < y?=w107:bool)
            n55 = case shown="False" w107 {
              tunnel: [-0.5 ("x") 0.0 ("x")] -> w108
              frame False {
              }
              frame True {
              }
            }
            n56 = call <vilib>:"WPI_MotorControlSetOutput.vi"("Output"=w108, "MotorControlDevRef"=w109) -> ("MotorControlDevRef"=w103:T4)  [unwired: 7 in, 2 out]
          }
        }
        frame #6 {
          w115 = T11 77 items=["Slot 0 - P"=1, "Slot 0 - I"=2, "Slot 0 - D"=3, "Slot 0 - F"=4, "Slot 0 - I Zone"=5, "Slot 0 - Ramp Rate"=6, "Slot 1 - P"=11, "Slot 1 - I"=12, "Slot 1 - D"=13, "Slot 1 - F"=14, "Slot 1 - I Zone"=15, "Slot 1 - Ramp Rate"=16, "Soft Limit - Forward"=21, "Soft Limit - Reverse"=22, "Soft Limit - Forward Enable"=23, "Soft Limit - Reverse Enable"=24, "On Boot - Brake Mode"=31, "On Boot - Limit Normally Closed - Forward"=32, "On Boot - Limit Normally Closed - Reverse"=33, "On Boot - Limit Disabled - Forward"=34, "On Boot - Limit Disabled - Reverse"=35, "Fault - Over Temp"=41, "Fault - Under Voltage"=42, "Fault - Forward Limit"=43, "Fault - Reverse Limit"=44, "Fault - Hardware Failure"=45, "Fault - Forward Soft Limit"=46, "Fault - Reverse Soft Limit"=47, "Sticky Fault - Over Temp"=48, "Sticky Fault - Under Voltage"=49, "Sticky Fault - Forward Limit"=50, "Sticky Fault - Reverse Limit"=51, "Sticky Fault - Forward Soft Limit"=52, "Sticky Fault - Reverse Soft Limit"=53, "Applied Throttle"=61, "Closed-Loop Error"=62, "Select Feedback Device"=63, "Reverse Closed-Loop Output"=64, "Mode Select"=65, "Profile Slot Select"=66, "Ramp Throttle"=67, "Reverse Feedback Sensor"=68, "Limit Switch Enabled"=69, "Limit Switch Closed - Forward"=70, "Limit Switch Closed - Reverse"=71, "Sensor Position"=73, "Sensor Velocity"=74, "Current"=75, "Brake is Enabled"=76, "Encoder Position"=77, "Encoder Velocity"=78, "Encoder Index Rise Events"=79, "Encoder A Pin State"=80, "Encoder B Pin State"=81, "Encoder Index Pin State"=82, "Analog In with Overflow"=83, "Analog In Velocity"=84, "Temperature"=85, "Battery Voltage"=86, "Reset Count"=87, "Reset Flags"=88, "Firmware Version"=89, "Settings Changed"=90, "Quad Filter Enable"=91, "Ignore Disable Broadcast"=92, "I Accumulator"=93, "Status 1 Frame Rate Ms"=94, "Status 2 Frame Rate Ms"=95, "Status 3 Frame Rate Ms"=96, "Status 4 Frame Rate Ms"=97, "Status 6 Frame Rate Ms"=98, "Status 7 Frame Rate Ms"=99, "Enable Index Pin Clear Position"=100, "Peak Positive Output"=104, "Nominal Positive Output"=105, "Peak Negative Output"=106, "Nominal Negative Output"=107, "Quad Index Pin Polarity"=108, "Status 8 Frame Rate Ms"=109, "Allow Position Overflow"=110, "Slot 0 - Allowable Closed-Loop Error"=111, "Number Potentiometer Turns"=112, "Encoder Codes Per Rev"=113, "Pulse Width Decoded Position"=114, "Analog Position"=115, "Voltage Compensation Rate (V/s)"=116, "Slot 1 - Allowable Closed-Loop Error"=117, "Motion Profile Has Underrun Err"=119, "Reserved 120"=120, "Legacy Control Mode"=121, "Motion Magic Acceleration"=122, "Motion Magic Cruise Velocity"=123, "Status 10 Frame Rate"=124, "Current Limit Threshold"=125, "CustomParam0"=137, "CustomParam1"=138, "PersStorageSaving"=139, "ClearPositionOnLimitF"=144, "ClearPositionOnLimitR"=145, "NominalBatteryVoltage"=146, "SampleVelocityPeriod"=147, "SampleVelocityWindow"=148] ("Parameter")
          n57 = Unbundle By Name(w113) -> ("CAN.Device Number"=w114:u8)
          n58 = call <vilib>:"WPI_CANTalonSRX_SetParameter.vi"("Value"=0.0, "Parameter"=w115, "Device ID (0)"=w114) -> ()  [unwired: 7 in, 2 out]
        }
        frame #7 {
          n59 = while {
            tunnel: w118 -> [w120]
            tunnel: [w119] -> w117
            stop <- w123 stop-if-true
            n60 = call <vilib>:"WPI_CANTalonSRX_GetStatus.vi"("CAN Talon SRX Ref"=w120) -> ("Talon SRX Status"=w126:T8, "CAN Talon SRX Ref"=w125:T4)  [unwired: 8 in, 1 out]
            n61 = Unbundle By Name(w126) -> ("Encoder Position"=w122:dbl)
            "Encoder Position 4" <- w122
            n62 = Greater?(x=-20000.0, y=w122) -> (0:w123:bool)
            n63 = case shown="False" w123 {
              tunnel: [0.3 ("x") 0.0 ("x")] -> w124
              frame False {
              }
              frame True {
              }
            }
            n64 = call <vilib>:"WPI_MotorControlSetOutput.vi"("Output"=w124, "MotorControlDevRef"=w125) -> ("MotorControlDevRef"=w119:T4)  [unwired: 7 in, 2 out]
          }
        }
        frame #8 {
          w131 = T11 77 items=["Slot 0 - P"=1, "Slot 0 - I"=2, "Slot 0 - D"=3, "Slot 0 - F"=4, "Slot 0 - I Zone"=5, "Slot 0 - Ramp Rate"=6, "Slot 1 - P"=11, "Slot 1 - I"=12, "Slot 1 - D"=13, "Slot 1 - F"=14, "Slot 1 - I Zone"=15, "Slot 1 - Ramp Rate"=16, "Soft Limit - Forward"=21, "Soft Limit - Reverse"=22, "Soft Limit - Forward Enable"=23, "Soft Limit - Reverse Enable"=24, "On Boot - Brake Mode"=31, "On Boot - Limit Normally Closed - Forward"=32, "On Boot - Limit Normally Closed - Reverse"=33, "On Boot - Limit Disabled - Forward"=34, "On Boot - Limit Disabled - Reverse"=35, "Fault - Over Temp"=41, "Fault - Under Voltage"=42, "Fault - Forward Limit"=43, "Fault - Reverse Limit"=44, "Fault - Hardware Failure"=45, "Fault - Forward Soft Limit"=46, "Fault - Reverse Soft Limit"=47, "Sticky Fault - Over Temp"=48, "Sticky Fault - Under Voltage"=49, "Sticky Fault - Forward Limit"=50, "Sticky Fault - Reverse Limit"=51, "Sticky Fault - Forward Soft Limit"=52, "Sticky Fault - Reverse Soft Limit"=53, "Applied Throttle"=61, "Closed-Loop Error"=62, "Select Feedback Device"=63, "Reverse Closed-Loop Output"=64, "Mode Select"=65, "Profile Slot Select"=66, "Ramp Throttle"=67, "Reverse Feedback Sensor"=68, "Limit Switch Enabled"=69, "Limit Switch Closed - Forward"=70, "Limit Switch Closed - Reverse"=71, "Sensor Position"=73, "Sensor Velocity"=74, "Current"=75, "Brake is Enabled"=76, "Encoder Position"=77, "Encoder Velocity"=78, "Encoder Index Rise Events"=79, "Encoder A Pin State"=80, "Encoder B Pin State"=81, "Encoder Index Pin State"=82, "Analog In with Overflow"=83, "Analog In Velocity"=84, "Temperature"=85, "Battery Voltage"=86, "Reset Count"=87, "Reset Flags"=88, "Firmware Version"=89, "Settings Changed"=90, "Quad Filter Enable"=91, "Ignore Disable Broadcast"=92, "I Accumulator"=93, "Status 1 Frame Rate Ms"=94, "Status 2 Frame Rate Ms"=95, "Status 3 Frame Rate Ms"=96, "Status 4 Frame Rate Ms"=97, "Status 6 Frame Rate Ms"=98, "Status 7 Frame Rate Ms"=99, "Enable Index Pin Clear Position"=100, "Peak Positive Output"=104, "Nominal Positive Output"=105, "Peak Negative Output"=106, "Nominal Negative Output"=107, "Quad Index Pin Polarity"=108, "Status 8 Frame Rate Ms"=109, "Allow Position Overflow"=110, "Slot 0 - Allowable Closed-Loop Error"=111, "Number Potentiometer Turns"=112, "Encoder Codes Per Rev"=113, "Pulse Width Decoded Position"=114, "Analog Position"=115, "Voltage Compensation Rate (V/s)"=116, "Slot 1 - Allowable Closed-Loop Error"=117, "Motion Profile Has Underrun Err"=119, "Reserved 120"=120, "Legacy Control Mode"=121, "Motion Magic Acceleration"=122, "Motion Magic Cruise Velocity"=123, "Status 10 Frame Rate"=124, "Current Limit Threshold"=125, "CustomParam0"=137, "CustomParam1"=138, "PersStorageSaving"=139, "ClearPositionOnLimitF"=144, "ClearPositionOnLimitR"=145, "NominalBatteryVoltage"=146, "SampleVelocityPeriod"=147, "SampleVelocityWindow"=148] ("Parameter")
          n65 = Unbundle By Name(w129) -> ("CAN.Device Number"=w130:u8)
          n66 = call <vilib>:"WPI_CANTalonSRX_SetParameter.vi"("Value"=0.0, "Parameter"=w131, "Device ID (0)"=w130) -> ()  [unwired: 7 in, 2 out]
        }
      }
    }
    frame "SHOOT" {
      n67 = call <vilib>:"WPI_CANTalonSRX_SetReference.vi"("error in (no error)"=w164, "Feedback Reference"=WPI_CANTalonSRX_APIFeedbackSelect."CTR Magnetic Enc (Relative)", "CAN Talon SRX Ref"=w165) -> ("error out"=w163:errorcluster, "CAN Talon SRX Ref"=w173:T4)  [unwired: 7 in]
      n68 = call <vilib>:"WPI_MotorControlSetOutput.vi"("error in (no error)"=w149, "Output"=0.75, "MotorControlDevRef"=w150) -> ("error out"=w146:errorcluster, "MotorControlDevRef"=w144:T4)  [unwired: 6 in, 1 out]
      n69 = call <vilib>:"WPI_CANTalonSRX_SetPID.vi"("CAN Talon SRX Ref"=w173, "P"=0.0, "I"=0.0, "D"=0.0, "error in (no error)"=w163, "F"=0.01, "I Zone"=0.0, "Ramp Rate"=0.0) -> ("CAN Talon SRX Ref"=w170:T4, "error out"=w162:errorcluster)  [unwired: 6 in]
      n70 = call <vilib>:"WPI_CANTalonSRX_ChangeMode.vi"("error in (no error)"=w162, "Output"=9800.0 ("y"), "Control Mode"=WPI_CANTalonSRX_APIControlMode."Speed", "CAN Talon SRX Ref"=w170) -> ("error out"=w161:errorcluster, "CAN Talon SRX Ref"=w166:T4)  [unwired: 6 in]
      n71 = call <vilib>:"WPI_CANTalonSRX_GetStatus.vi"("error in (no error)"=w161, "CAN Talon SRX Ref"=w166) -> ("error out"=w147:errorcluster)  [unwired: 7 in, 2 out]
      n72 = Merge Errors(w147, w146) -> (w145:errorcluster)
      n73 = call <vilib>:"WPI_RobotDriveDelayAndUpdateSafety.vi"("error in (no error)"=w145, "Delay (s)"=10.0, "RobotDriveDevRef"=w159) -> ("error out"=w143:errorcluster, "RobotDriveDevRef 2"=w160:T9)  [unwired: 7 in]
      n74 = call <vilib>:"WPI_MotorControlSetOutput.vi"("error in (no error)"=w143, "Output"=0.0, "MotorControlDevRef"=w144) -> ()  [unwired: 6 in, 3 out]
      n75 = call-poly <vilib>:"WPI_RobotDriveArcadeDrive.vi"("error in (no error)"=w143, "Y axis value"=0.0, "X axis value"=0.4, "RobotDriveDevRef"=w160) -> ("error out"=w156:errorcluster, "RobotDriveDevRef"=w157:T9)  [unwired: 5 in, 1 out]
      n76 = call <vilib>:"WPI_RobotDriveDelayAndUpdateSafety.vi"("error in (no error)"=w156, "Delay (s)"=1.0, "RobotDriveDevRef"=w157) -> ("error out"=w136:errorcluster, "RobotDriveDevRef 2"=w135:T9)  [unwired: 7 in]
      n77 = call-poly <vilib>:"WPI_RobotDriveArcadeDrive.vi"("error in (no error)"=w136, "Y axis value"=-0.6, "X axis value"=0.0, "RobotDriveDevRef"=w135) -> ("error out"=w139:errorcluster, "RobotDriveDevRef"=w140:T9)  [unwired: 5 in, 1 out]
      n78 = call <vilib>:"WPI_RobotDriveDelayAndUpdateSafety.vi"("error in (no error)"=w139, "Delay (s)"=3.0, "RobotDriveDevRef"=w140) -> ("error out"=w133:errorcluster, "RobotDriveDevRef 2"=w134:T9)  [unwired: 7 in]
      n79 = call-poly <vilib>:"WPI_RobotDriveArcadeDrive.vi"("error in (no error)"=w133, "Y axis value"=0.0, "X axis value"=0.0, "RobotDriveDevRef"=w134) -> ()  [unwired: 5 in, 3 out]
    }
    frame "SHOOTRED" {
      # "SHOOTRED"
      n80 = call <vilib>:"WPI_CANTalonSRX_SetReference.vi"("error in (no error)"=w230, "Feedback Reference"=WPI_CANTalonSRX_APIFeedbackSelect."CTR Magnetic Enc (Relative)", "CAN Talon SRX Ref"=w231) -> ("error out"=w229:errorcluster, "CAN Talon SRX Ref"=w239:T4)  [unwired: 7 in]
      n81 = call <vilib>:"WPI_MotorControlSetOutput.vi"("error in (no error)"=w217, "Output"=0.75, "MotorControlDevRef"=w218) -> ("error out"=w214:errorcluster, "MotorControlDevRef"=w212:T4)  [unwired: 6 in, 1 out]
      n82 = call <vilib>:"WPI_CANTalonSRX_SetPID.vi"("CAN Talon SRX Ref"=w239, "P"=0.0, "I"=0.0, "D"=0.0, "error in (no error)"=w229, "F"=0.01, "I Zone"=0.0, "Ramp Rate"=0.0) -> ("CAN Talon SRX Ref"=w236:T4, "error out"=w228:errorcluster)  [unwired: 6 in]
      n83 = call <vilib>:"WPI_CANTalonSRX_ChangeMode.vi"("error in (no error)"=w228, "Output"=9800.0 ("y"), "Control Mode"=WPI_CANTalonSRX_APIControlMode."Speed", "CAN Talon SRX Ref"=w236) -> ("error out"=w227:errorcluster, "CAN Talon SRX Ref"=w232:T4)  [unwired: 6 in]
      n84 = call <vilib>:"WPI_CANTalonSRX_GetStatus.vi"("error in (no error)"=w227, "CAN Talon SRX Ref"=w232) -> ("error out"=w215:errorcluster, "CAN Talon SRX Ref"=w197:T4)  [unwired: 7 in, 1 out]
      n85 = Merge Errors(w215, w214) -> (w213:errorcluster)
      n86 = call <vilib>:"WPI_RobotDriveDelayAndUpdateSafety.vi"("error in (no error)"=w213, "Delay (s)"=10.0, "RobotDriveDevRef"=w225) -> ("error out"=w196:errorcluster, "RobotDriveDevRef 2"=w226:T9)  [unwired: 7 in]
      n87 = call <vilib>:"WPI_CANTalonSRX_ChangeMode.vi"("error in (no error)"=w196, "Output"=0.0 ("y"), "Control Mode"=WPI_CANTalonSRX_APIControlMode."Speed", "CAN Talon SRX Ref"=w197) -> ("error out"=w198:errorcluster, "CAN Talon SRX Ref"=w199:T4)  [unwired: 6 in]
      n88 = call <vilib>:"WPI_MotorControlSetOutput.vi"("error in (no error)"=w196, "Output"=0.0, "MotorControlDevRef"=w212) -> ("error out"=w194:errorcluster)  [unwired: 6 in, 2 out]
      n89 = call <vilib>:"WPI_CANTalonSRX_GetStatus.vi"("error in (no error)"=w198, "CAN Talon SRX Ref"=w199) -> ("error out"=w195:errorcluster)  [unwired: 7 in, 2 out]
      n90 = Merge Errors(w195, w194) -> (w193:errorcluster)
      n91 = call <vilib>:"WPI_RobotDriveTankDrive.vi"("error in (no error)"=w193, "Right axis value"=0.6 ("Y axis value"), "Left axis value"=0.6, "RobotDriveDevRef"=w226) -> ("error out"=w223:errorcluster, "RobotDriveDevRef"=w224:T9)  [unwired: 5 in, 1 out]
      n92 = call <vilib>:"WPI_RobotDriveDelayAndUpdateSafety.vi"("error in (no error)"=w223, "Delay (s)"=0.25, "RobotDriveDevRef"=w224) -> ("error out"=w205:errorcluster, "RobotDriveDevRef 2"=w204:T9)  [unwired: 7 in]
      n93 = call-poly <vilib>:"WPI_RobotDriveArcadeDrive.vi"("error in (no error)"=w205, "Y axis value"=0.0, "X axis value"=-0.8, "RobotDriveDevRef"=w204) -> ("error out"=w208:errorcluster, "RobotDriveDevRef"=w209:T9)  [unwired: 5 in, 1 out]
      n94 = call <vilib>:"WPI_RobotDriveDelayAndUpdateSafety.vi"("error in (no error)"=w208, "Delay (s)"=0.5, "RobotDriveDevRef"=w209) -> ("error out"=w202:errorcluster, "RobotDriveDevRef 2"=w203:T9)  [unwired: 7 in]
      n95 = call-poly <vilib>:"WPI_RobotDriveArcadeDrive.vi"("error in (no error)"=w202, "Y axis value"=-0.5, "X axis value"=-0.55, "RobotDriveDevRef"=w203) -> ("error out"=w191:errorcluster, "RobotDriveDevRef"=w192:T9)  [unwired: 5 in, 1 out]
      n96 = call <vilib>:"WPI_RobotDriveDelayAndUpdateSafety.vi"("error in (no error)"=w191, "Delay (s)"=1.0, "RobotDriveDevRef"=w192) -> ("error out"=w189:errorcluster, "RobotDriveDevRef 2"=w188:T9)  [unwired: 7 in]
      n97 = call-poly <vilib>:"WPI_RobotDriveArcadeDrive.vi"("error in (no error)"=w189, "Y axis value"=-0.5 ("X axis value"), "RobotDriveDevRef"=w188) -> ("error out"=w183:errorcluster, "RobotDriveDevRef"=w184:T9)  [unwired: 6 in, 1 out]
      n98 = call <vilib>:"WPI_RobotDriveDelayAndUpdateSafety.vi"("error in (no error)"=w183, "Delay (s)"=2.0, "RobotDriveDevRef"=w184) -> ("error out"=w180:errorcluster, "RobotDriveDevRef 2"=w181:T9)  [unwired: 7 in]
      n99 = call-poly <vilib>:"WPI_RobotDriveArcadeDrive.vi"("error in (no error)"=w180, "Y axis value"=0.0, "X axis value"=0.0, "RobotDriveDevRef"=w181) -> ()  [unwired: 5 in, 3 out]
    }
    frame "TEST" {
      n100 = flat-sequence {
        tunnel: w247 -> [w249]
        tunnel: [w249] -> w245
        tunnel: [w248] -> w244
        tunnel: w246 -> [w255]
        tunnel: w245 -> [w254]
        tunnel: w244 -> [w253]
        frame #0 {
          w251 = T11 77 items=["Slot 0 - P"=1, "Slot 0 - I"=2, "Slot 0 - D"=3, "Slot 0 - F"=4, "Slot 0 - I Zone"=5, "Slot 0 - Ramp Rate"=6, "Slot 1 - P"=11, "Slot 1 - I"=12, "Slot 1 - D"=13, "Slot 1 - F"=14, "Slot 1 - I Zone"=15, "Slot 1 - Ramp Rate"=16, "Soft Limit - Forward"=21, "Soft Limit - Reverse"=22, "Soft Limit - Forward Enable"=23, "Soft Limit - Reverse Enable"=24, "On Boot - Brake Mode"=31, "On Boot - Limit Normally Closed - Forward"=32, "On Boot - Limit Normally Closed - Reverse"=33, "On Boot - Limit Disabled - Forward"=34, "On Boot - Limit Disabled - Reverse"=35, "Fault - Over Temp"=41, "Fault - Under Voltage"=42, "Fault - Forward Limit"=43, "Fault - Reverse Limit"=44, "Fault - Hardware Failure"=45, "Fault - Forward Soft Limit"=46, "Fault - Reverse Soft Limit"=47, "Sticky Fault - Over Temp"=48, "Sticky Fault - Under Voltage"=49, "Sticky Fault - Forward Limit"=50, "Sticky Fault - Reverse Limit"=51, "Sticky Fault - Forward Soft Limit"=52, "Sticky Fault - Reverse Soft Limit"=53, "Applied Throttle"=61, "Closed-Loop Error"=62, "Select Feedback Device"=63, "Reverse Closed-Loop Output"=64, "Mode Select"=65, "Profile Slot Select"=66, "Ramp Throttle"=67, "Reverse Feedback Sensor"=68, "Limit Switch Enabled"=69, "Limit Switch Closed - Forward"=70, "Limit Switch Closed - Reverse"=71, "Sensor Position"=73, "Sensor Velocity"=74, "Current"=75, "Brake is Enabled"=76, "Encoder Position"=77, "Encoder Velocity"=78, "Encoder Index Rise Events"=79, "Encoder A Pin State"=80, "Encoder B Pin State"=81, "Encoder Index Pin State"=82, "Analog In with Overflow"=83, "Analog In Velocity"=84, "Temperature"=85, "Battery Voltage"=86, "Reset Count"=87, "Reset Flags"=88, "Firmware Version"=89, "Settings Changed"=90, "Quad Filter Enable"=91, "Ignore Disable Broadcast"=92, "I Accumulator"=93, "Status 1 Frame Rate Ms"=94, "Status 2 Frame Rate Ms"=95, "Status 3 Frame Rate Ms"=96, "Status 4 Frame Rate Ms"=97, "Status 6 Frame Rate Ms"=98, "Status 7 Frame Rate Ms"=99, "Enable Index Pin Clear Position"=100, "Peak Positive Output"=104, "Nominal Positive Output"=105, "Peak Negative Output"=106, "Nominal Negative Output"=107, "Quad Index Pin Polarity"=108, "Status 8 Frame Rate Ms"=109, "Allow Position Overflow"=110, "Slot 0 - Allowable Closed-Loop Error"=111, "Number Potentiometer Turns"=112, "Encoder Codes Per Rev"=113, "Pulse Width Decoded Position"=114, "Analog Position"=115, "Voltage Compensation Rate (V/s)"=116, "Slot 1 - Allowable Closed-Loop Error"=117, "Motion Profile Has Underrun Err"=119, "Reserved 120"=120, "Legacy Control Mode"=121, "Motion Magic Acceleration"=122, "Motion Magic Cruise Velocity"=123, "Status 10 Frame Rate"=124, "Current Limit Threshold"=125, "CustomParam0"=137, "CustomParam1"=138, "PersStorageSaving"=139, "ClearPositionOnLimitF"=144, "ClearPositionOnLimitR"=145, "NominalBatteryVoltage"=146, "SampleVelocityPeriod"=147, "SampleVelocityWindow"=148] ("Parameter")
          n101 = Unbundle By Name(w249) -> ("CAN.Device Number"=w252:u8)
          n102 = call <vilib>:"WPI_CANTalonSRX_SetParameter.vi"("Value"=0.0, "Parameter"=w251, "Device ID (0)"=w252) -> ("error out"=w248:errorcluster)  [unwired: 7 in, 1 out]
        }
        frame #1 {
          n103 = while {
            tunnel: w255 -> [w258]
            tunnel: w254 -> [w257]
            tunnel: w253 -> [w256]
            stop <- w260 stop-if-true
            n104 = Greater?(x=w258, y=10000.0) -> (0:w260:bool)
            n105 = Select(t=0.0, s=w260, f=0.2) -> (s? t:f=w261:dbl)
            n106 = call <vilib>:"WPI_MotorControlSetOutput.vi"("error in (no error)"=w256, "Output"=w261, "MotorControlDevRef"=w257) -> ()  [unwired: 6 in, 3 out]
          }
        }
      }
    }
    frame "TEST1" {
      n107 = call <vilib>:"WPI_MotorControlSetOutput.vi"("Output"=0.2, "MotorControlDevRef"=w264) -> ()  [unwired: 7 in, 3 out]
    }
    frame "MIDDLE" {
      n108 = call-poly <vilib>:"WPI_RobotDriveArcadeDrive.vi"("error in (no error)"=w295, "Y axis value"=0.45, "RobotDriveDevRef"=w296) -> ("error out"=w292:errorcluster, "RobotDriveDevRef"=w293:T9)  [unwired: 6 in, 1 out]
      n109 = call <vilib>:"WPI_RobotDriveDelayAndUpdateSafety.vi"("error in (no error)"=w292, "Delay (s)"=2.0, "RobotDriveDevRef"=w293) -> ("error out"=w290:errorcluster, "RobotDriveDevRef 2"=w289:T9)  [unwired: 7 in]
      n110 = call-poly <vilib>:"WPI_RobotDriveArcadeDrive.vi"("error in (no error)"=w290, "Y axis value"=0.0, "RobotDriveDevRef"=w289) -> ("error out"=w286:errorcluster, "RobotDriveDevRef"=w287:T9)  [unwired: 6 in, 1 out]
      n111 = call <vilib>:"WPI_RobotDriveDelayAndUpdateSafety.vi"("error in (no error)"=w286, "Delay (s)"=0.5, "RobotDriveDevRef"=w287) -> ("error out"=w284:errorcluster, "RobotDriveDevRef 2"=w282:T9)  [unwired: 7 in]
      n112 = call <vilib>:"WPI_MotorControlSetOutput.vi"("error in (no error)"=w284, "Output"=-0.7, "MotorControlDevRef"=w283) -> ("error out"=w281:errorcluster, "MotorControlDevRef"=w277:T4)  [unwired: 6 in, 1 out]
      n113 = call <vilib>:"WPI_RobotDriveDelayAndUpdateSafety.vi"("error in (no error)"=w281, "Delay (s)"=1.5, "RobotDriveDevRef"=w282) -> ("error out"=w278:errorcluster, "RobotDriveDevRef 2"=w275:T9)  [unwired: 7 in]
      n114 = call <vilib>:"WPI_MotorControlSetOutput.vi"("error in (no error)"=w278, "Output"=0.0, "MotorControlDevRef"=w277) -> ("error out"=w274:errorcluster)  [unwired: 6 in, 2 out]
      n115 = call-poly <vilib>:"WPI_RobotDriveArcadeDrive.vi"("error in (no error)"=w274, "Y axis value"=-0.4, "RobotDriveDevRef"=w275) -> ("error out"=w271:errorcluster, "RobotDriveDevRef"=w272:T9)  [unwired: 6 in, 1 out]
      n116 = call <vilib>:"WPI_RobotDriveDelayAndUpdateSafety.vi"("error in (no error)"=w271, "Delay (s)"=2.0, "RobotDriveDevRef"=w272) -> ("error out"=w268:errorcluster, "RobotDriveDevRef 2"=w269:T9)  [unwired: 7 in]
      n117 = call-poly <vilib>:"WPI_RobotDriveArcadeDrive.vi"("error in (no error)"=w268, "Y axis value"=0.0, "X axis value"=0.0, "RobotDriveDevRef"=w269) -> ()  [unwired: 5 in, 3 out]
    }
    frame "RIGHTSIDE" {
      # "RIGHTSIDE"
      n118 = call-poly <vilib>:"WPI_RobotDriveArcadeDrive.vi"("error in (no error)"=w298, "Y axis value"=0.59, "RobotDriveDevRef"=w299) -> ("error out"=w338:errorcluster, "RobotDriveDevRef"=w339:T9)  [unwired: 6 in, 1 out]
      n119 = call <vilib>:"WPI_RobotDriveDelayAndUpdateSafety.vi"("error in (no error)"=w338, "Delay (s)"=1.8, "RobotDriveDevRef"=w339) -> ("error out"=w334:errorcluster, "RobotDriveDevRef 2"=w335:T9)  [unwired: 7 in]
      n120 = call-poly <vilib>:"WPI_RobotDriveArcadeDrive.vi"("error in (no error)"=w334, "X axis value"=0.36, "RobotDriveDevRef"=w335) -> ("error out"=w331:errorcluster, "RobotDriveDevRef"=w332:T9)  [unwired: 6 in, 1 out]
      n121 = call <vilib>:"WPI_RobotDriveDelayAndUpdateSafety.vi"("error in (no error)"=w331, "Delay (s)"=1.0, "RobotDriveDevRef"=w332) -> ("error out"=w328:errorcluster, "RobotDriveDevRef 2"=w329:T9)  [unwired: 7 in]
      n122 = call-poly <vilib>:"WPI_RobotDriveArcadeDrive.vi"("error in (no error)"=w328, "Y axis value"=0.5, "RobotDriveDevRef"=w329) -> ("error out"=w325:errorcluster, "RobotDriveDevRef"=w326:T9)  [unwired: 6 in, 1 out]
      n123 = call <vilib>:"WPI_RobotDriveDelayAndUpdateSafety.vi"("error in (no error)"=w325, "Delay (s)"=2.3, "RobotDriveDevRef"=w326) -> ("error out"=w322:errorcluster, "RobotDriveDevRef 2"=w323:T9)  [unwired: 7 in]
      n124 = call-poly <vilib>:"WPI_RobotDriveArcadeDrive.vi"("error in (no error)"=w322, "Y axis value"=0.0, "RobotDriveDevRef"=w323) -> ("error out"=w319:errorcluster, "RobotDriveDevRef"=w320:T9)  [unwired: 6 in, 1 out]
      n125 = call <vilib>:"WPI_RobotDriveDelayAndUpdateSafety.vi"("error in (no error)"=w319, "Delay (s)"=0.5, "RobotDriveDevRef"=w320) -> ("error out"=w317:errorcluster, "RobotDriveDevRef 2"=w315:T9)  [unwired: 7 in]
      n126 = call <vilib>:"WPI_MotorControlSetOutput.vi"("error in (no error)"=w317, "Output"=-0.7, "MotorControlDevRef"=w297) -> ("error out"=w314:errorcluster, "MotorControlDevRef"=w303:T4)  [unwired: 6 in, 1 out]
      n127 = call <vilib>:"WPI_RobotDriveDelayAndUpdateSafety.vi"("error in (no error)"=w314, "Delay (s)"=1.5, "RobotDriveDevRef"=w315) -> ("error out"=w302:errorcluster, "RobotDriveDevRef 2"=w312:T9)  [unwired: 7 in]
      n128 = call <vilib>:"WPI_MotorControlSetOutput.vi"("error in (no error)"=w302, "Output"=0.0, "MotorControlDevRef"=w303) -> ("error out"=w300:errorcluster)  [unwired: 6 in, 2 out]
      n129 = call-poly <vilib>:"WPI_RobotDriveArcadeDrive.vi"("error in (no error)"=w300, "Y axis value"=-0.4, "RobotDriveDevRef"=w312) -> ("error out"=w309:errorcluster, "RobotDriveDevRef"=w310:T9)  [unwired: 6 in, 1 out]
      n130 = call <vilib>:"WPI_RobotDriveDelayAndUpdateSafety.vi"("error in (no error)"=w309, "Delay (s)"=2.0, "RobotDriveDevRef"=w310) -> ("error out"=w307:errorcluster, "RobotDriveDevRef 2"=w306:T9)  [unwired: 7 in]
      n131 = call-poly <vilib>:"WPI_RobotDriveArcadeDrive.vi"("error in (no error)"=w307, "Y axis value"=0.0, "X axis value"=0.0, "RobotDriveDevRef"=w306) -> ()  [unwired: 5 in, 3 out]
    }
    frame "LEFTSIDE" {
      n132 = call-poly <vilib>:"WPI_RobotDriveArcadeDrive.vi"("error in (no error)"=w381, "Y axis value"=0.6, "RobotDriveDevRef"=w382) -> ("error out"=w379:errorcluster, "RobotDriveDevRef"=w380:T9)  [unwired: 6 in, 1 out]
      n133 = call <vilib>:"WPI_RobotDriveDelayAndUpdateSafety.vi"("error in (no error)"=w379, "Delay (s)"=2.0, "RobotDriveDevRef"=w380) -> ("error out"=w375:errorcluster, "RobotDriveDevRef 2"=w376:T9)  [unwired: 7 in]
      n134 = call-poly <vilib>:"WPI_RobotDriveArcadeDrive.vi"("error in (no error)"=w375, "X axis value"=-0.45, "RobotDriveDevRef"=w376) -> ("error out"=w372:errorcluster, "RobotDriveDevRef"=w373:T9)  [unwired: 6 in, 1 out]
      n135 = call <vilib>:"WPI_RobotDriveDelayAndUpdateSafety.vi"("error in (no error)"=w372, "Delay (s)"=1.0, "RobotDriveDevRef"=w373) -> ("error out"=w369:errorcluster, "RobotDriveDevRef 2"=w370:T9)  [unwired: 7 in]
      n136 = call-poly <vilib>:"WPI_RobotDriveArcadeDrive.vi"("error in (no error)"=w369, "Y axis value"=0.52, "RobotDriveDevRef"=w370) -> ("error out"=w366:errorcluster, "RobotDriveDevRef"=w367:T9)  [unwired: 6 in, 1 out]
      n137 = call <vilib>:"WPI_RobotDriveDelayAndUpdateSafety.vi"("error in (no error)"=w366, "Delay (s)"=2.25, "RobotDriveDevRef"=w367) -> ("error out"=w363:errorcluster, "RobotDriveDevRef 2"=w364:T9)  [unwired: 7 in]
      n138 = call-poly <vilib>:"WPI_RobotDriveArcadeDrive.vi"("error in (no error)"=w363, "Y axis value"=0.0, "RobotDriveDevRef"=w364) -> ("error out"=w360:errorcluster, "RobotDriveDevRef"=w361:T9)  [unwired: 6 in, 1 out]
      n139 = call <vilib>:"WPI_RobotDriveDelayAndUpdateSafety.vi"("error in (no error)"=w360, "Delay (s)"=0.5, "RobotDriveDevRef"=w361) -> ("error out"=w357:errorcluster, "RobotDriveDevRef 2"=w355:T9)  [unwired: 7 in]
      n140 = call <vilib>:"WPI_MotorControlSetOutput.vi"("error in (no error)"=w357, "Output"=-0.7, "MotorControlDevRef"=w358) -> ("error out"=w354:errorcluster, "MotorControlDevRef"=w343:T4)  [unwired: 6 in, 1 out]
      n141 = call <vilib>:"WPI_RobotDriveDelayAndUpdateSafety.vi"("error in (no error)"=w354, "Delay (s)"=1.5, "RobotDriveDevRef"=w355) -> ("error out"=w342:errorcluster, "RobotDriveDevRef 2"=w352:T9)  [unwired: 7 in]
      n142 = call <vilib>:"WPI_MotorControlSetOutput.vi"("error in (no error)"=w342, "Output"=0.0, "MotorControlDevRef"=w343) -> ("error out"=w340:errorcluster)  [unwired: 6 in, 2 out]
      n143 = call-poly <vilib>:"WPI_RobotDriveArcadeDrive.vi"("error in (no error)"=w340, "Y axis value"=-0.4, "RobotDriveDevRef"=w352) -> ("error out"=w349:errorcluster, "RobotDriveDevRef"=w350:T9)  [unwired: 6 in, 1 out]
      n144 = call <vilib>:"WPI_RobotDriveDelayAndUpdateSafety.vi"("error in (no error)"=w349, "Delay (s)"=2.0, "RobotDriveDevRef"=w350) -> ("error out"=w347:errorcluster, "RobotDriveDevRef 2"=w346:T9)  [unwired: 7 in]
      n145 = call-poly <vilib>:"WPI_RobotDriveArcadeDrive.vi"("error in (no error)"=w347, "Y axis value"=0.0, "X axis value"=0.0, "RobotDriveDevRef"=w346) -> ()  [unwired: 5 in, 3 out]
    }
    frame "A" {
      n146 = flat-sequence {
        tunnel: w389 -> [w403]
        tunnel: [w403] -> w400
        tunnel: w384 -> [w401]
        tunnel: [w401] -> w383
        tunnel: w400 -> [w412]
        tunnel: [w411] -> w399
        tunnel: [w410] -> w398
        tunnel: w383 -> [w409]
        tunnel: w399 -> [w435]
        tunnel: w398 -> [w434]
        tunnel: [w435] -> w397
        tunnel: [w434] -> w396
        tunnel: [w443] -> w386
        tunnel: [w442] -> w385
        tunnel: w396 -> [w444]
        tunnel: w397 -> [w445]
        tunnel: [w468] -> w395
        tunnel: [w467] -> w394
        tunnel: w385 -> [w467]
        tunnel: w386 -> [w468]
        tunnel: w395 -> [w476]
        tunnel: w394 -> [w477]
        tunnel: [w476] -> w393
        tunnel: [w475] -> w391
        tunnel: w393 -> [w488]
        tunnel: [w488] -> w392
        tunnel: w391 -> [w492]
        tunnel: [w492] -> w390
        tunnel: w392 -> [w498]
        tunnel: w390 -> [w499]
        tunnel: [w497] -> w387
        tunnel: [w496] -> w388
        tunnel: w387 -> [w522]
        tunnel: w388 -> [w524]
        frame #0 {
          w404 = T11 77 items=["Slot 0 - P"=1, "Slot 0 - I"=2, "Slot 0 - D"=3, "Slot 0 - F"=4, "Slot 0 - I Zone"=5, "Slot 0 - Ramp Rate"=6, "Slot 1 - P"=11, "Slot 1 - I"=12, "Slot 1 - D"=13, "Slot 1 - F"=14, "Slot 1 - I Zone"=15, "Slot 1 - Ramp Rate"=16, "Soft Limit - Forward"=21, "Soft Limit - Reverse"=22, "Soft Limit - Forward Enable"=23, "Soft Limit - Reverse Enable"=24, "On Boot - Brake Mode"=31, "On Boot - Limit Normally Closed - Forward"=32, "On Boot - Limit Normally Closed - Reverse"=33, "On Boot - Limit Disabled - Forward"=34, "On Boot - Limit Disabled - Reverse"=35, "Fault - Over Temp"=41, "Fault - Under Voltage"=42, "Fault - Forward Limit"=43, "Fault - Reverse Limit"=44, "Fault - Hardware Failure"=45, "Fault - Forward Soft Limit"=46, "Fault - Reverse Soft Limit"=47, "Sticky Fault - Over Temp"=48, "Sticky Fault - Under Voltage"=49, "Sticky Fault - Forward Limit"=50, "Sticky Fault - Reverse Limit"=51, "Sticky Fault - Forward Soft Limit"=52, "Sticky Fault - Reverse Soft Limit"=53, "Applied Throttle"=61, "Closed-Loop Error"=62, "Select Feedback Device"=63, "Reverse Closed-Loop Output"=64, "Mode Select"=65, "Profile Slot Select"=66, "Ramp Throttle"=67, "Reverse Feedback Sensor"=68, "Limit Switch Enabled"=69, "Limit Switch Closed - Forward"=70, "Limit Switch Closed - Reverse"=71, "Sensor Position"=73, "Sensor Velocity"=74, "Current"=75, "Brake is Enabled"=76, "Encoder Position"=77, "Encoder Velocity"=78, "Encoder Index Rise Events"=79, "Encoder A Pin State"=80, "Encoder B Pin State"=81, "Encoder Index Pin State"=82, "Analog In with Overflow"=83, "Analog In Velocity"=84, "Temperature"=85, "Battery Voltage"=86, "Reset Count"=87, "Reset Flags"=88, "Firmware Version"=89, "Settings Changed"=90, "Quad Filter Enable"=91, "Ignore Disable Broadcast"=92, "I Accumulator"=93, "Status 1 Frame Rate Ms"=94, "Status 2 Frame Rate Ms"=95, "Status 3 Frame Rate Ms"=96, "Status 4 Frame Rate Ms"=97, "Status 6 Frame Rate Ms"=98, "Status 7 Frame Rate Ms"=99, "Enable Index Pin Clear Position"=100, "Peak Positive Output"=104, "Nominal Positive Output"=105, "Peak Negative Output"=106, "Nominal Negative Output"=107, "Quad Index Pin Polarity"=108, "Status 8 Frame Rate Ms"=109, "Allow Position Overflow"=110, "Slot 0 - Allowable Closed-Loop Error"=111, "Number Potentiometer Turns"=112, "Encoder Codes Per Rev"=113, "Pulse Width Decoded Position"=114, "Analog Position"=115, "Voltage Compensation Rate (V/s)"=116, "Slot 1 - Allowable Closed-Loop Error"=117, "Motion Profile Has Underrun Err"=119, "Reserved 120"=120, "Legacy Control Mode"=121, "Motion Magic Acceleration"=122, "Motion Magic Cruise Velocity"=123, "Status 10 Frame Rate"=124, "Current Limit Threshold"=125, "CustomParam0"=137, "CustomParam1"=138, "PersStorageSaving"=139, "ClearPositionOnLimitF"=144, "ClearPositionOnLimitR"=145, "NominalBatteryVoltage"=146, "SampleVelocityPeriod"=147, "SampleVelocityWindow"=148] ("Parameter")
          w407 = T11 77 items=["Slot 0 - P"=1, "Slot 0 - I"=2, "Slot 0 - D"=3, "Slot 0 - F"=4, "Slot 0 - I Zone"=5, "Slot 0 - Ramp Rate"=6, "Slot 1 - P"=11, "Slot 1 - I"=12, "Slot 1 - D"=13, "Slot 1 - F"=14, "Slot 1 - I Zone"=15, "Slot 1 - Ramp Rate"=16, "Soft Limit - Forward"=21, "Soft Limit - Reverse"=22, "Soft Limit - Forward Enable"=23, "Soft Limit - Reverse Enable"=24, "On Boot - Brake Mode"=31, "On Boot - Limit Normally Closed - Forward"=32, "On Boot - Limit Normally Closed - Reverse"=33, "On Boot - Limit Disabled - Forward"=34, "On Boot - Limit Disabled - Reverse"=35, "Fault - Over Temp"=41, "Fault - Under Voltage"=42, "Fault - Forward Limit"=43, "Fault - Reverse Limit"=44, "Fault - Hardware Failure"=45, "Fault - Forward Soft Limit"=46, "Fault - Reverse Soft Limit"=47, "Sticky Fault - Over Temp"=48, "Sticky Fault - Under Voltage"=49, "Sticky Fault - Forward Limit"=50, "Sticky Fault - Reverse Limit"=51, "Sticky Fault - Forward Soft Limit"=52, "Sticky Fault - Reverse Soft Limit"=53, "Applied Throttle"=61, "Closed-Loop Error"=62, "Select Feedback Device"=63, "Reverse Closed-Loop Output"=64, "Mode Select"=65, "Profile Slot Select"=66, "Ramp Throttle"=67, "Reverse Feedback Sensor"=68, "Limit Switch Enabled"=69, "Limit Switch Closed - Forward"=70, "Limit Switch Closed - Reverse"=71, "Sensor Position"=73, "Sensor Velocity"=74, "Current"=75, "Brake is Enabled"=76, "Encoder Position"=77, "Encoder Velocity"=78, "Encoder Index Rise Events"=79, "Encoder A Pin State"=80, "Encoder B Pin State"=81, "Encoder Index Pin State"=82, "Analog In with Overflow"=83, "Analog In Velocity"=84, "Temperature"=85, "Battery Voltage"=86, "Reset Count"=87, "Reset Flags"=88, "Firmware Version"=89, "Settings Changed"=90, "Quad Filter Enable"=91, "Ignore Disable Broadcast"=92, "I Accumulator"=93, "Status 1 Frame Rate Ms"=94, "Status 2 Frame Rate Ms"=95, "Status 3 Frame Rate Ms"=96, "Status 4 Frame Rate Ms"=97, "Status 6 Frame Rate Ms"=98, "Status 7 Frame Rate Ms"=99, "Enable Index Pin Clear Position"=100, "Peak Positive Output"=104, "Nominal Positive Output"=105, "Peak Negative Output"=106, "Nominal Negative Output"=107, "Quad Index Pin Polarity"=108, "Status 8 Frame Rate Ms"=109, "Allow Position Overflow"=110, "Slot 0 - Allowable Closed-Loop Error"=111, "Number Potentiometer Turns"=112, "Encoder Codes Per Rev"=113, "Pulse Width Decoded Position"=114, "Analog Position"=115, "Voltage Compensation Rate (V/s)"=116, "Slot 1 - Allowable Closed-Loop Error"=117, "Motion Profile Has Underrun Err"=119, "Reserved 120"=120, "Legacy Control Mode"=121, "Motion Magic Acceleration"=122, "Motion Magic Cruise Velocity"=123, "Status 10 Frame Rate"=124, "Current Limit Threshold"=125, "CustomParam0"=137, "CustomParam1"=138, "PersStorageSaving"=139, "ClearPositionOnLimitF"=144, "ClearPositionOnLimitR"=145, "NominalBatteryVoltage"=146, "SampleVelocityPeriod"=147, "SampleVelocityWindow"=148] ("Parameter")
          n147 = Unbundle By Name(w403) -> ("CAN.Device Number"=w402:u8)
          n148 = Unbundle By Name(w401) -> ("CAN.Device Number"=w408:u8)
          n149 = call <vilib>:"WPI_CANTalonSRX_SetParameter.vi"("Value"=0.0, "Parameter"=w404, "Device ID (0)"=w402) -> ()  [unwired: 7 in, 2 out]
          n150 = call <vilib>:"WPI_CANTalonSRX_SetParameter.vi"("Value"=0.0, "Parameter"=w407, "Device ID (0)"=w408) -> ()  [unwired: 7 in, 2 out]
        }
        frame #1 {
          n151 = while {
            tunnel: w412 -> [w425]
            tunnel: [w424] -> w410
            tunnel: [w423] -> w411
            tunnel: w409 -> [w413]
            stop <- w416 stop-if-true
            n152 = call <vilib>:"WPI_CANTalonSRX_GetStatus.vi"("CAN Talon SRX Ref"=w413) -> ("Talon SRX Status"=w421:T8, "CAN Talon SRX Ref"=w417:T4)  [unwired: 8 in, 1 out]
            n153 = call <vilib>:"WPI_CANTalonSRX_GetStatus.vi"("CAN Talon SRX Ref"=w425) -> ("Talon SRX Status"=w426:T8, "CAN Talon SRX Ref"=w427:T4)  [unwired: 8 in, 1 out]
            n154 = Unbundle By Name(w421) -> ("Encoder Position"=w420:dbl)
            "Encoder Position 7" <- w420
            n155 = Unbundle By Name(w426) -> ("Encoder Position"=w428:dbl)
            "Encoder Position 6" <- w428
            n156 = Less?(x=-2256.0, y=w420) -> (x < y?=w414:bool)
            n157 = Greater?(x=5325.0, y=w428) -> (0:w415:bool)
            n158 = And(x=w414, y=w415) -> (x .and. y?=w416:bool)
            n159 = case shown="True" w414 {
              tunnel: [0.0 ("Output") 0.2 ("Output")] -> w418
              frame False {
              }
              frame True {
              }
            }
            n160 = case shown="True" w415 {
              tunnel: [0.0 ("Output") 0.2 ("Output")] -> w422
              frame False {
              }
              frame True {
              }
            }
            n161 = call <vilib>:"WPI_MotorControlSetOutput.vi"("Output"=w418, "MotorControlDevRef"=w417) -> ("MotorControlDevRef"=w423:T4)  [unwired: 7 in, 2 out]
            n162 = call <vilib>:"WPI_MotorControlSetOutput.vi"("Output"=w422, "MotorControlDevRef"=w427) -> ("MotorControlDevRef"=w424:T4)  [unwired: 7 in, 2 out]
          }
        }
        frame #2 {
          w440 = T11 77 items=["Slot 0 - P"=1, "Slot 0 - I"=2, "Slot 0 - D"=3, "Slot 0 - F"=4, "Slot 0 - I Zone"=5, "Slot 0 - Ramp Rate"=6, "Slot 1 - P"=11, "Slot 1 - I"=12, "Slot 1 - D"=13, "Slot 1 - F"=14, "Slot 1 - I Zone"=15, "Slot 1 - Ramp Rate"=16, "Soft Limit - Forward"=21, "Soft Limit - Reverse"=22, "Soft Limit - Forward Enable"=23, "Soft Limit - Reverse Enable"=24, "On Boot - Brake Mode"=31, "On Boot - Limit Normally Closed - Forward"=32, "On Boot - Limit Normally Closed - Reverse"=33, "On Boot - Limit Disabled - Forward"=34, "On Boot - Limit Disabled - Reverse"=35, "Fault - Over Temp"=41, "Fault - Under Voltage"=42, "Fault - Forward Limit"=43, "Fault - Reverse Limit"=44, "Fault - Hardware Failure"=45, "Fault - Forward Soft Limit"=46, "Fault - Reverse Soft Limit"=47, "Sticky Fault - Over Temp"=48, "Sticky Fault - Under Voltage"=49, "Sticky Fault - Forward Limit"=50, "Sticky Fault - Reverse Limit"=51, "Sticky Fault - Forward Soft Limit"=52, "Sticky Fault - Reverse Soft Limit"=53, "Applied Throttle"=61, "Closed-Loop Error"=62, "Select Feedback Device"=63, "Reverse Closed-Loop Output"=64, "Mode Select"=65, "Profile Slot Select"=66, "Ramp Throttle"=67, "Reverse Feedback Sensor"=68, "Limit Switch Enabled"=69, "Limit Switch Closed - Forward"=70, "Limit Switch Closed - Reverse"=71, "Sensor Position"=73, "Sensor Velocity"=74, "Current"=75, "Brake is Enabled"=76, "Encoder Position"=77, "Encoder Velocity"=78, "Encoder Index Rise Events"=79, "Encoder A Pin State"=80, "Encoder B Pin State"=81, "Encoder Index Pin State"=82, "Analog In with Overflow"=83, "Analog In Velocity"=84, "Temperature"=85, "Battery Voltage"=86, "Reset Count"=87, "Reset Flags"=88, "Firmware Version"=89, "Settings Changed"=90, "Quad Filter Enable"=91, "Ignore Disable Broadcast"=92, "I Accumulator"=93, "Status 1 Frame Rate Ms"=94, "Status 2 Frame Rate Ms"=95, "Status 3 Frame Rate Ms"=96, "Status 4 Frame Rate Ms"=97, "Status 6 Frame Rate Ms"=98, "Status 7 Frame Rate Ms"=99, "Enable Index Pin Clear Position"=100, "Peak Positive Output"=104, "Nominal Positive Output"=105, "Peak Negative Output"=106, "Nominal Negative Output"=107, "Quad Index Pin Polarity"=108, "Status 8 Frame Rate Ms"=109, "Allow Position Overflow"=110, "Slot 0 - Allowable Closed-Loop Error"=111, "Number Potentiometer Turns"=112, "Encoder Codes Per Rev"=113, "Pulse Width Decoded Position"=114, "Analog Position"=115, "Voltage Compensation Rate (V/s)"=116, "Slot 1 - Allowable Closed-Loop Error"=117, "Motion Profile Has Underrun Err"=119, "Reserved 120"=120, "Legacy Control Mode"=121, "Motion Magic Acceleration"=122, "Motion Magic Cruise Velocity"=123, "Status 10 Frame Rate"=124, "Current Limit Threshold"=125, "CustomParam0"=137, "CustomParam1"=138, "PersStorageSaving"=139, "ClearPositionOnLimitF"=144, "ClearPositionOnLimitR"=145, "NominalBatteryVoltage"=146, "SampleVelocityPeriod"=147, "SampleVelocityWindow"=148] ("Parameter")
          w437 = T11 77 items=["Slot 0 - P"=1, "Slot 0 - I"=2, "Slot 0 - D"=3, "Slot 0 - F"=4, "Slot 0 - I Zone"=5, "Slot 0 - Ramp Rate"=6, "Slot 1 - P"=11, "Slot 1 - I"=12, "Slot 1 - D"=13, "Slot 1 - F"=14, "Slot 1 - I Zone"=15, "Slot 1 - Ramp Rate"=16, "Soft Limit - Forward"=21, "Soft Limit - Reverse"=22, "Soft Limit - Forward Enable"=23, "Soft Limit - Reverse Enable"=24, "On Boot - Brake Mode"=31, "On Boot - Limit Normally Closed - Forward"=32, "On Boot - Limit Normally Closed - Reverse"=33, "On Boot - Limit Disabled - Forward"=34, "On Boot - Limit Disabled - Reverse"=35, "Fault - Over Temp"=41, "Fault - Under Voltage"=42, "Fault - Forward Limit"=43, "Fault - Reverse Limit"=44, "Fault - Hardware Failure"=45, "Fault - Forward Soft Limit"=46, "Fault - Reverse Soft Limit"=47, "Sticky Fault - Over Temp"=48, "Sticky Fault - Under Voltage"=49, "Sticky Fault - Forward Limit"=50, "Sticky Fault - Reverse Limit"=51, "Sticky Fault - Forward Soft Limit"=52, "Sticky Fault - Reverse Soft Limit"=53, "Applied Throttle"=61, "Closed-Loop Error"=62, "Select Feedback Device"=63, "Reverse Closed-Loop Output"=64, "Mode Select"=65, "Profile Slot Select"=66, "Ramp Throttle"=67, "Reverse Feedback Sensor"=68, "Limit Switch Enabled"=69, "Limit Switch Closed - Forward"=70, "Limit Switch Closed - Reverse"=71, "Sensor Position"=73, "Sensor Velocity"=74, "Current"=75, "Brake is Enabled"=76, "Encoder Position"=77, "Encoder Velocity"=78, "Encoder Index Rise Events"=79, "Encoder A Pin State"=80, "Encoder B Pin State"=81, "Encoder Index Pin State"=82, "Analog In with Overflow"=83, "Analog In Velocity"=84, "Temperature"=85, "Battery Voltage"=86, "Reset Count"=87, "Reset Flags"=88, "Firmware Version"=89, "Settings Changed"=90, "Quad Filter Enable"=91, "Ignore Disable Broadcast"=92, "I Accumulator"=93, "Status 1 Frame Rate Ms"=94, "Status 2 Frame Rate Ms"=95, "Status 3 Frame Rate Ms"=96, "Status 4 Frame Rate Ms"=97, "Status 6 Frame Rate Ms"=98, "Status 7 Frame Rate Ms"=99, "Enable Index Pin Clear Position"=100, "Peak Positive Output"=104, "Nominal Positive Output"=105, "Peak Negative Output"=106, "Nominal Negative Output"=107, "Quad Index Pin Polarity"=108, "Status 8 Frame Rate Ms"=109, "Allow Position Overflow"=110, "Slot 0 - Allowable Closed-Loop Error"=111, "Number Potentiometer Turns"=112, "Encoder Codes Per Rev"=113, "Pulse Width Decoded Position"=114, "Analog Position"=115, "Voltage Compensation Rate (V/s)"=116, "Slot 1 - Allowable Closed-Loop Error"=117, "Motion Profile Has Underrun Err"=119, "Reserved 120"=120, "Legacy Control Mode"=121, "Motion Magic Acceleration"=122, "Motion Magic Cruise Velocity"=123, "Status 10 Frame Rate"=124, "Current Limit Threshold"=125, "CustomParam0"=137, "CustomParam1"=138, "PersStorageSaving"=139, "ClearPositionOnLimitF"=144, "ClearPositionOnLimitR"=145, "NominalBatteryVoltage"=146, "SampleVelocityPeriod"=147, "SampleVelocityWindow"=148] ("Parameter")
          n163 = Unbundle By Name(w434) -> ("CAN.Device Number"=w441:u8)
          n164 = Unbundle By Name(w435) -> ("CAN.Device Number"=w436:u8)
          n165 = call <vilib>:"WPI_CANTalonSRX_SetParameter.vi"("Value"=0.0, "Parameter"=w440, "Device ID (0)"=w441) -> ()  [unwired: 7 in, 2 out]
          n166 = call <vilib>:"WPI_CANTalonSRX_SetParameter.vi"("Value"=0.0, "Parameter"=w437, "Device ID (0)"=w436) -> ()  [unwired: 7 in, 2 out]
        }
        frame #3 {
          n167 = while {
            tunnel: w445 -> [w462]
            tunnel: w444 -> [w451]
            tunnel: [w447] -> w443
            tunnel: [w446] -> w442
            stop <- w448 stop-if-true
            n168 = call <vilib>:"WPI_CANTalonSRX_GetStatus.vi"("CAN Talon SRX Ref"=w462) -> ("Talon SRX Status"=w461:T8, "CAN Talon SRX Ref"=w460:T4)  [unwired: 8 in, 1 out]
            n169 = call <vilib>:"WPI_CANTalonSRX_GetStatus.vi"("CAN Talon SRX Ref"=w451) -> ("Talon SRX Status"=w452:T8, "CAN Talon SRX Ref"=w453:T4)  [unwired: 8 in, 1 out]
            n170 = Unbundle By Name(w461) -> ("Encoder Position"=w459:dbl)
            n171 = Unbundle By Name(w452) -> ("Encoder Position"=w454:dbl)
            n172 = Greater?(x=1980.0, y=w459) -> (0:w449:bool)
            n173 = Less?(x=-4125.0, y=w454) -> (x < y?=w450:bool)
            n174 = case shown="False" w449 {
              tunnel: [-0.3 ("Output") 0.0 ("Output")] -> w457
              frame False {
              }
              frame True {
              }
            }
            n175 = case shown="False" w450 {
              tunnel: [-0.3 ("Output") 0.0 ("Output")] -> w456
              frame False {
              }
              frame True {
              }
            }
            n176 = And(x=w449, y=w450) -> (x .and. y?=w448:bool)
            n177 = call <vilib>:"WPI_MotorControlSetOutput.vi"("Output"=w457, "MotorControlDevRef"=w460) -> ("MotorControlDevRef"=w446:T4)  [unwired: 7 in, 2 out]
            n178 = call <vilib>:"WPI_MotorControlSetOutput.vi"("Output"=w456, "MotorControlDevRef"=w453) -> ("MotorControlDevRef"=w447:T4)  [unwired: 7 in, 2 out]
          }
        }
        frame #4 {
          w473 = T11 77 items=["Slot 0 - P"=1, "Slot 0 - I"=2, "Slot 0 - D"=3, "Slot 0 - F"=4, "Slot 0 - I Zone"=5, "Slot 0 - Ramp Rate"=6, "Slot 1 - P"=11, "Slot 1 - I"=12, "Slot 1 - D"=13, "Slot 1 - F"=14, "Slot 1 - I Zone"=15, "Slot 1 - Ramp Rate"=16, "Soft Limit - Forward"=21, "Soft Limit - Reverse"=22, "Soft Limit - Forward Enable"=23, "Soft Limit - Reverse Enable"=24, "On Boot - Brake Mode"=31, "On Boot - Limit Normally Closed - Forward"=32, "On Boot - Limit Normally Closed - Reverse"=33, "On Boot - Limit Disabled - Forward"=34, "On Boot - Limit Disabled - Reverse"=35, "Fault - Over Temp"=41, "Fault - Under Voltage"=42, "Fault - Forward Limit"=43, "Fault - Reverse Limit"=44, "Fault - Hardware Failure"=45, "Fault - Forward Soft Limit"=46, "Fault - Reverse Soft Limit"=47, "Sticky Fault - Over Temp"=48, "Sticky Fault - Under Voltage"=49, "Sticky Fault - Forward Limit"=50, "Sticky Fault - Reverse Limit"=51, "Sticky Fault - Forward Soft Limit"=52, "Sticky Fault - Reverse Soft Limit"=53, "Applied Throttle"=61, "Closed-Loop Error"=62, "Select Feedback Device"=63, "Reverse Closed-Loop Output"=64, "Mode Select"=65, "Profile Slot Select"=66, "Ramp Throttle"=67, "Reverse Feedback Sensor"=68, "Limit Switch Enabled"=69, "Limit Switch Closed - Forward"=70, "Limit Switch Closed - Reverse"=71, "Sensor Position"=73, "Sensor Velocity"=74, "Current"=75, "Brake is Enabled"=76, "Encoder Position"=77, "Encoder Velocity"=78, "Encoder Index Rise Events"=79, "Encoder A Pin State"=80, "Encoder B Pin State"=81, "Encoder Index Pin State"=82, "Analog In with Overflow"=83, "Analog In Velocity"=84, "Temperature"=85, "Battery Voltage"=86, "Reset Count"=87, "Reset Flags"=88, "Firmware Version"=89, "Settings Changed"=90, "Quad Filter Enable"=91, "Ignore Disable Broadcast"=92, "I Accumulator"=93, "Status 1 Frame Rate Ms"=94, "Status 2 Frame Rate Ms"=95, "Status 3 Frame Rate Ms"=96, "Status 4 Frame Rate Ms"=97, "Status 6 Frame Rate Ms"=98, "Status 7 Frame Rate Ms"=99, "Enable Index Pin Clear Position"=100, "Peak Positive Output"=104, "Nominal Positive Output"=105, "Peak Negative Output"=106, "Nominal Negative Output"=107, "Quad Index Pin Polarity"=108, "Status 8 Frame Rate Ms"=109, "Allow Position Overflow"=110, "Slot 0 - Allowable Closed-Loop Error"=111, "Number Potentiometer Turns"=112, "Encoder Codes Per Rev"=113, "Pulse Width Decoded Position"=114, "Analog Position"=115, "Voltage Compensation Rate (V/s)"=116, "Slot 1 - Allowable Closed-Loop Error"=117, "Motion Profile Has Underrun Err"=119, "Reserved 120"=120, "Legacy Control Mode"=121, "Motion Magic Acceleration"=122, "Motion Magic Cruise Velocity"=123, "Status 10 Frame Rate"=124, "Current Limit Threshold"=125, "CustomParam0"=137, "CustomParam1"=138, "PersStorageSaving"=139, "ClearPositionOnLimitF"=144, "ClearPositionOnLimitR"=145, "NominalBatteryVoltage"=146, "SampleVelocityPeriod"=147, "SampleVelocityWindow"=148] ("Parameter")
          w470 = T11 77 items=["Slot 0 - P"=1, "Slot 0 - I"=2, "Slot 0 - D"=3, "Slot 0 - F"=4, "Slot 0 - I Zone"=5, "Slot 0 - Ramp Rate"=6, "Slot 1 - P"=11, "Slot 1 - I"=12, "Slot 1 - D"=13, "Slot 1 - F"=14, "Slot 1 - I Zone"=15, "Slot 1 - Ramp Rate"=16, "Soft Limit - Forward"=21, "Soft Limit - Reverse"=22, "Soft Limit - Forward Enable"=23, "Soft Limit - Reverse Enable"=24, "On Boot - Brake Mode"=31, "On Boot - Limit Normally Closed - Forward"=32, "On Boot - Limit Normally Closed - Reverse"=33, "On Boot - Limit Disabled - Forward"=34, "On Boot - Limit Disabled - Reverse"=35, "Fault - Over Temp"=41, "Fault - Under Voltage"=42, "Fault - Forward Limit"=43, "Fault - Reverse Limit"=44, "Fault - Hardware Failure"=45, "Fault - Forward Soft Limit"=46, "Fault - Reverse Soft Limit"=47, "Sticky Fault - Over Temp"=48, "Sticky Fault - Under Voltage"=49, "Sticky Fault - Forward Limit"=50, "Sticky Fault - Reverse Limit"=51, "Sticky Fault - Forward Soft Limit"=52, "Sticky Fault - Reverse Soft Limit"=53, "Applied Throttle"=61, "Closed-Loop Error"=62, "Select Feedback Device"=63, "Reverse Closed-Loop Output"=64, "Mode Select"=65, "Profile Slot Select"=66, "Ramp Throttle"=67, "Reverse Feedback Sensor"=68, "Limit Switch Enabled"=69, "Limit Switch Closed - Forward"=70, "Limit Switch Closed - Reverse"=71, "Sensor Position"=73, "Sensor Velocity"=74, "Current"=75, "Brake is Enabled"=76, "Encoder Position"=77, "Encoder Velocity"=78, "Encoder Index Rise Events"=79, "Encoder A Pin State"=80, "Encoder B Pin State"=81, "Encoder Index Pin State"=82, "Analog In with Overflow"=83, "Analog In Velocity"=84, "Temperature"=85, "Battery Voltage"=86, "Reset Count"=87, "Reset Flags"=88, "Firmware Version"=89, "Settings Changed"=90, "Quad Filter Enable"=91, "Ignore Disable Broadcast"=92, "I Accumulator"=93, "Status 1 Frame Rate Ms"=94, "Status 2 Frame Rate Ms"=95, "Status 3 Frame Rate Ms"=96, "Status 4 Frame Rate Ms"=97, "Status 6 Frame Rate Ms"=98, "Status 7 Frame Rate Ms"=99, "Enable Index Pin Clear Position"=100, "Peak Positive Output"=104, "Nominal Positive Output"=105, "Peak Negative Output"=106, "Nominal Negative Output"=107, "Quad Index Pin Polarity"=108, "Status 8 Frame Rate Ms"=109, "Allow Position Overflow"=110, "Slot 0 - Allowable Closed-Loop Error"=111, "Number Potentiometer Turns"=112, "Encoder Codes Per Rev"=113, "Pulse Width Decoded Position"=114, "Analog Position"=115, "Voltage Compensation Rate (V/s)"=116, "Slot 1 - Allowable Closed-Loop Error"=117, "Motion Profile Has Underrun Err"=119, "Reserved 120"=120, "Legacy Control Mode"=121, "Motion Magic Acceleration"=122, "Motion Magic Cruise Velocity"=123, "Status 10 Frame Rate"=124, "Current Limit Threshold"=125, "CustomParam0"=137, "CustomParam1"=138, "PersStorageSaving"=139, "ClearPositionOnLimitF"=144, "ClearPositionOnLimitR"=145, "NominalBatteryVoltage"=146, "SampleVelocityPeriod"=147, "SampleVelocityWindow"=148] ("Parameter")
          n179 = Unbundle By Name(w468) -> ("CAN.Device Number"=w474:u8)
          n180 = Unbundle By Name(w467) -> ("CAN.Device Number"=w469:u8)
          n181 = call <vilib>:"WPI_CANTalonSRX_SetParameter.vi"("Value"=0.0, "Parameter"=w473, "Device ID (0)"=w474) -> ()  [unwired: 7 in, 2 out]
          n182 = call <vilib>:"WPI_CANTalonSRX_SetParameter.vi"("Value"=0.0, "Parameter"=w470, "Device ID (0)"=w469) -> ()  [unwired: 7 in, 2 out]
        }
        frame #5 {
          n183 = while {
            tunnel: w477 -> [w485]
            tunnel: [w478] -> w475
            stop <- w479 stop-if-true
            n184 = call <vilib>:"WPI_CANTalonSRX_GetStatus.vi"("CAN Talon SRX Ref"=w485) -> ("Talon SRX Status"=w484:T8, "CAN Talon SRX Ref"=w480:T4)  [unwired: 8 in, 1 out]
            n185 = Unbundle By Name(w484) -> ("Encoder Position"=w483:dbl)
            n186 = Less?(x=-1500.0, y=w483) -> (x < y?=w479:bool)
            n187 = case shown="False" w479 {
              tunnel: [-0.3 ("Output") 0.0 ("Output")] -> w481
              frame False {
              }
              frame True {
              }
            }
            n188 = call <vilib>:"WPI_MotorControlSetOutput.vi"("Output"=w481, "MotorControlDevRef"=w480) -> ("MotorControlDevRef"=w478:T4)  [unwired: 7 in, 2 out]
          }
        }
        frame #6 {
          w490 = T11 77 items=["Slot 0 - P"=1, "Slot 0 - I"=2, "Slot 0 - D"=3, "Slot 0 - F"=4, "Slot 0 - I Zone"=5, "Slot 0 - Ramp Rate"=6, "Slot 1 - P"=11, "Slot 1 - I"=12, "Slot 1 - D"=13, "Slot 1 - F"=14, "Slot 1 - I Zone"=15, "Slot 1 - Ramp Rate"=16, "Soft Limit - Forward"=21, "Soft Limit - Reverse"=22, "Soft Limit - Forward Enable"=23, "Soft Limit - Reverse Enable"=24, "On Boot - Brake Mode"=31, "On Boot - Limit Normally Closed - Forward"=32, "On Boot - Limit Normally Closed - Reverse"=33, "On Boot - Limit Disabled - Forward"=34, "On Boot - Limit Disabled - Reverse"=35, "Fault - Over Temp"=41, "Fault - Under Voltage"=42, "Fault - Forward Limit"=43, "Fault - Reverse Limit"=44, "Fault - Hardware Failure"=45, "Fault - Forward Soft Limit"=46, "Fault - Reverse Soft Limit"=47, "Sticky Fault - Over Temp"=48, "Sticky Fault - Under Voltage"=49, "Sticky Fault - Forward Limit"=50, "Sticky Fault - Reverse Limit"=51, "Sticky Fault - Forward Soft Limit"=52, "Sticky Fault - Reverse Soft Limit"=53, "Applied Throttle"=61, "Closed-Loop Error"=62, "Select Feedback Device"=63, "Reverse Closed-Loop Output"=64, "Mode Select"=65, "Profile Slot Select"=66, "Ramp Throttle"=67, "Reverse Feedback Sensor"=68, "Limit Switch Enabled"=69, "Limit Switch Closed - Forward"=70, "Limit Switch Closed - Reverse"=71, "Sensor Position"=73, "Sensor Velocity"=74, "Current"=75, "Brake is Enabled"=76, "Encoder Position"=77, "Encoder Velocity"=78, "Encoder Index Rise Events"=79, "Encoder A Pin State"=80, "Encoder B Pin State"=81, "Encoder Index Pin State"=82, "Analog In with Overflow"=83, "Analog In Velocity"=84, "Temperature"=85, "Battery Voltage"=86, "Reset Count"=87, "Reset Flags"=88, "Firmware Version"=89, "Settings Changed"=90, "Quad Filter Enable"=91, "Ignore Disable Broadcast"=92, "I Accumulator"=93, "Status 1 Frame Rate Ms"=94, "Status 2 Frame Rate Ms"=95, "Status 3 Frame Rate Ms"=96, "Status 4 Frame Rate Ms"=97, "Status 6 Frame Rate Ms"=98, "Status 7 Frame Rate Ms"=99, "Enable Index Pin Clear Position"=100, "Peak Positive Output"=104, "Nominal Positive Output"=105, "Peak Negative Output"=106, "Nominal Negative Output"=107, "Quad Index Pin Polarity"=108, "Status 8 Frame Rate Ms"=109, "Allow Position Overflow"=110, "Slot 0 - Allowable Closed-Loop Error"=111, "Number Potentiometer Turns"=112, "Encoder Codes Per Rev"=113, "Pulse Width Decoded Position"=114, "Analog Position"=115, "Voltage Compensation Rate (V/s)"=116, "Slot 1 - Allowable Closed-Loop Error"=117, "Motion Profile Has Underrun Err"=119, "Reserved 120"=120, "Legacy Control Mode"=121, "Motion Magic Acceleration"=122, "Motion Magic Cruise Velocity"=123, "Status 10 Frame Rate"=124, "Current Limit Threshold"=125, "CustomParam0"=137, "CustomParam1"=138, "PersStorageSaving"=139, "ClearPositionOnLimitF"=144, "ClearPositionOnLimitR"=145, "NominalBatteryVoltage"=146, "SampleVelocityPeriod"=147, "SampleVelocityWindow"=148] ("Parameter")
          w494 = T11 77 items=["Slot 0 - P"=1, "Slot 0 - I"=2, "Slot 0 - D"=3, "Slot 0 - F"=4, "Slot 0 - I Zone"=5, "Slot 0 - Ramp Rate"=6, "Slot 1 - P"=11, "Slot 1 - I"=12, "Slot 1 - D"=13, "Slot 1 - F"=14, "Slot 1 - I Zone"=15, "Slot 1 - Ramp Rate"=16, "Soft Limit - Forward"=21, "Soft Limit - Reverse"=22, "Soft Limit - Forward Enable"=23, "Soft Limit - Reverse Enable"=24, "On Boot - Brake Mode"=31, "On Boot - Limit Normally Closed - Forward"=32, "On Boot - Limit Normally Closed - Reverse"=33, "On Boot - Limit Disabled - Forward"=34, "On Boot - Limit Disabled - Reverse"=35, "Fault - Over Temp"=41, "Fault - Under Voltage"=42, "Fault - Forward Limit"=43, "Fault - Reverse Limit"=44, "Fault - Hardware Failure"=45, "Fault - Forward Soft Limit"=46, "Fault - Reverse Soft Limit"=47, "Sticky Fault - Over Temp"=48, "Sticky Fault - Under Voltage"=49, "Sticky Fault - Forward Limit"=50, "Sticky Fault - Reverse Limit"=51, "Sticky Fault - Forward Soft Limit"=52, "Sticky Fault - Reverse Soft Limit"=53, "Applied Throttle"=61, "Closed-Loop Error"=62, "Select Feedback Device"=63, "Reverse Closed-Loop Output"=64, "Mode Select"=65, "Profile Slot Select"=66, "Ramp Throttle"=67, "Reverse Feedback Sensor"=68, "Limit Switch Enabled"=69, "Limit Switch Closed - Forward"=70, "Limit Switch Closed - Reverse"=71, "Sensor Position"=73, "Sensor Velocity"=74, "Current"=75, "Brake is Enabled"=76, "Encoder Position"=77, "Encoder Velocity"=78, "Encoder Index Rise Events"=79, "Encoder A Pin State"=80, "Encoder B Pin State"=81, "Encoder Index Pin State"=82, "Analog In with Overflow"=83, "Analog In Velocity"=84, "Temperature"=85, "Battery Voltage"=86, "Reset Count"=87, "Reset Flags"=88, "Firmware Version"=89, "Settings Changed"=90, "Quad Filter Enable"=91, "Ignore Disable Broadcast"=92, "I Accumulator"=93, "Status 1 Frame Rate Ms"=94, "Status 2 Frame Rate Ms"=95, "Status 3 Frame Rate Ms"=96, "Status 4 Frame Rate Ms"=97, "Status 6 Frame Rate Ms"=98, "Status 7 Frame Rate Ms"=99, "Enable Index Pin Clear Position"=100, "Peak Positive Output"=104, "Nominal Positive Output"=105, "Peak Negative Output"=106, "Nominal Negative Output"=107, "Quad Index Pin Polarity"=108, "Status 8 Frame Rate Ms"=109, "Allow Position Overflow"=110, "Slot 0 - Allowable Closed-Loop Error"=111, "Number Potentiometer Turns"=112, "Encoder Codes Per Rev"=113, "Pulse Width Decoded Position"=114, "Analog Position"=115, "Voltage Compensation Rate (V/s)"=116, "Slot 1 - Allowable Closed-Loop Error"=117, "Motion Profile Has Underrun Err"=119, "Reserved 120"=120, "Legacy Control Mode"=121, "Motion Magic Acceleration"=122, "Motion Magic Cruise Velocity"=123, "Status 10 Frame Rate"=124, "Current Limit Threshold"=125, "CustomParam0"=137, "CustomParam1"=138, "PersStorageSaving"=139, "ClearPositionOnLimitF"=144, "ClearPositionOnLimitR"=145, "NominalBatteryVoltage"=146, "SampleVelocityPeriod"=147, "SampleVelocityWindow"=148] ("Parameter")
          n189 = Unbundle By Name(w492) -> ("CAN.Device Number"=w493:u8)
          n190 = Unbundle By Name(w488) -> ("CAN.Device Number"=w491:u8)
          n191 = call <vilib>:"WPI_CANTalonSRX_SetParameter.vi"("Value"=0.0, "Parameter"=w494, "Device ID (0)"=w493) -> ()  [unwired: 7 in, 2 out]
          n192 = call <vilib>:"WPI_CANTalonSRX_SetParameter.vi"("Value"=0.0, "Parameter"=w490, "Device ID (0)"=w491) -> ()  [unwired: 7 in, 2 out]
        }
        frame #7 {
          n193 = while {
            tunnel: w499 -> [w516]
            tunnel: w498 -> [w505]
            tunnel: [w501] -> w497
            tunnel: [w500] -> w496
            stop <- w502 stop-if-true
            n194 = call <vilib>:"WPI_CANTalonSRX_GetStatus.vi"("CAN Talon SRX Ref"=w516) -> ("Talon SRX Status"=w515:T8, "CAN Talon SRX Ref"=w514:T4)  [unwired: 8 in, 1 out]
            n195 = call <vilib>:"WPI_CANTalonSRX_GetStatus.vi"("CAN Talon SRX Ref"=w505) -> ("Talon SRX Status"=w506:T8, "CAN Talon SRX Ref"=w507:T4)  [unwired: 8 in, 1 out]
            n196 = Unbundle By Name(w515) -> ("Encoder Position"=w513:dbl)
            n197 = Unbundle By Name(w506) -> ("Encoder Position"=w508:dbl)
            n198 = Less?(x=-4500.0, y=w513) -> (x < y?=w503:bool)
            n199 = Greater?(x=9375.0, y=w508) -> (0:w504:bool)
            n200 = case shown="False" w503 {
              tunnel: [-0.3 ("Output") 0.0 ("Output")] -> w511
              frame False {
              }
              frame True {
              }
            }
            n201 = case shown="False" w504 {
              tunnel: [-0.3 ("Output") 0.0 ("Output")] -> w510
              frame False {
              }
              frame True {
              }
            }
            n202 = And(x=w503, y=w504) -> (x .and. y?=w502:bool)
            n203 = call <vilib>:"WPI_MotorControlSetOutput.vi"("Output"=w511, "MotorControlDevRef"=w514) -> ("MotorControlDevRef"=w500:T4)  [unwired: 7 in, 2 out]
            n204 = call <vilib>:"WPI_MotorControlSetOutput.vi"("Output"=w510, "MotorControlDevRef"=w507) -> ("MotorControlDevRef"=w501:T4)  [unwired: 7 in, 2 out]
          }
        }
        frame #8 {
          w526 = T11 77 items=["Slot 0 - P"=1, "Slot 0 - I"=2, "Slot 0 - D"=3, "Slot 0 - F"=4, "Slot 0 - I Zone"=5, "Slot 0 - Ramp Rate"=6, "Slot 1 - P"=11, "Slot 1 - I"=12, "Slot 1 - D"=13, "Slot 1 - F"=14, "Slot 1 - I Zone"=15, "Slot 1 - Ramp Rate"=16, "Soft Limit - Forward"=21, "Soft Limit - Reverse"=22, "Soft Limit - Forward Enable"=23, "Soft Limit - Reverse Enable"=24, "On Boot - Brake Mode"=31, "On Boot - Limit Normally Closed - Forward"=32, "On Boot - Limit Normally Closed - Reverse"=33, "On Boot - Limit Disabled - Forward"=34, "On Boot - Limit Disabled - Reverse"=35, "Fault - Over Temp"=41, "Fault - Under Voltage"=42, "Fault - Forward Limit"=43, "Fault - Reverse Limit"=44, "Fault - Hardware Failure"=45, "Fault - Forward Soft Limit"=46, "Fault - Reverse Soft Limit"=47, "Sticky Fault - Over Temp"=48, "Sticky Fault - Under Voltage"=49, "Sticky Fault - Forward Limit"=50, "Sticky Fault - Reverse Limit"=51, "Sticky Fault - Forward Soft Limit"=52, "Sticky Fault - Reverse Soft Limit"=53, "Applied Throttle"=61, "Closed-Loop Error"=62, "Select Feedback Device"=63, "Reverse Closed-Loop Output"=64, "Mode Select"=65, "Profile Slot Select"=66, "Ramp Throttle"=67, "Reverse Feedback Sensor"=68, "Limit Switch Enabled"=69, "Limit Switch Closed - Forward"=70, "Limit Switch Closed - Reverse"=71, "Sensor Position"=73, "Sensor Velocity"=74, "Current"=75, "Brake is Enabled"=76, "Encoder Position"=77, "Encoder Velocity"=78, "Encoder Index Rise Events"=79, "Encoder A Pin State"=80, "Encoder B Pin State"=81, "Encoder Index Pin State"=82, "Analog In with Overflow"=83, "Analog In Velocity"=84, "Temperature"=85, "Battery Voltage"=86, "Reset Count"=87, "Reset Flags"=88, "Firmware Version"=89, "Settings Changed"=90, "Quad Filter Enable"=91, "Ignore Disable Broadcast"=92, "I Accumulator"=93, "Status 1 Frame Rate Ms"=94, "Status 2 Frame Rate Ms"=95, "Status 3 Frame Rate Ms"=96, "Status 4 Frame Rate Ms"=97, "Status 6 Frame Rate Ms"=98, "Status 7 Frame Rate Ms"=99, "Enable Index Pin Clear Position"=100, "Peak Positive Output"=104, "Nominal Positive Output"=105, "Peak Negative Output"=106, "Nominal Negative Output"=107, "Quad Index Pin Polarity"=108, "Status 8 Frame Rate Ms"=109, "Allow Position Overflow"=110, "Slot 0 - Allowable Closed-Loop Error"=111, "Number Potentiometer Turns"=112, "Encoder Codes Per Rev"=113, "Pulse Width Decoded Position"=114, "Analog Position"=115, "Voltage Compensation Rate (V/s)"=116, "Slot 1 - Allowable Closed-Loop Error"=117, "Motion Profile Has Underrun Err"=119, "Reserved 120"=120, "Legacy Control Mode"=121, "Motion Magic Acceleration"=122, "Motion Magic Cruise Velocity"=123, "Status 10 Frame Rate"=124, "Current Limit Threshold"=125, "CustomParam0"=137, "CustomParam1"=138, "PersStorageSaving"=139, "ClearPositionOnLimitF"=144, "ClearPositionOnLimitR"=145, "NominalBatteryVoltage"=146, "SampleVelocityPeriod"=147, "SampleVelocityWindow"=148] ("Parameter")
          w527 = T11 77 items=["Slot 0 - P"=1, "Slot 0 - I"=2, "Slot 0 - D"=3, "Slot 0 - F"=4, "Slot 0 - I Zone"=5, "Slot 0 - Ramp Rate"=6, "Slot 1 - P"=11, "Slot 1 - I"=12, "Slot 1 - D"=13, "Slot 1 - F"=14, "Slot 1 - I Zone"=15, "Slot 1 - Ramp Rate"=16, "Soft Limit - Forward"=21, "Soft Limit - Reverse"=22, "Soft Limit - Forward Enable"=23, "Soft Limit - Reverse Enable"=24, "On Boot - Brake Mode"=31, "On Boot - Limit Normally Closed - Forward"=32, "On Boot - Limit Normally Closed - Reverse"=33, "On Boot - Limit Disabled - Forward"=34, "On Boot - Limit Disabled - Reverse"=35, "Fault - Over Temp"=41, "Fault - Under Voltage"=42, "Fault - Forward Limit"=43, "Fault - Reverse Limit"=44, "Fault - Hardware Failure"=45, "Fault - Forward Soft Limit"=46, "Fault - Reverse Soft Limit"=47, "Sticky Fault - Over Temp"=48, "Sticky Fault - Under Voltage"=49, "Sticky Fault - Forward Limit"=50, "Sticky Fault - Reverse Limit"=51, "Sticky Fault - Forward Soft Limit"=52, "Sticky Fault - Reverse Soft Limit"=53, "Applied Throttle"=61, "Closed-Loop Error"=62, "Select Feedback Device"=63, "Reverse Closed-Loop Output"=64, "Mode Select"=65, "Profile Slot Select"=66, "Ramp Throttle"=67, "Reverse Feedback Sensor"=68, "Limit Switch Enabled"=69, "Limit Switch Closed - Forward"=70, "Limit Switch Closed - Reverse"=71, "Sensor Position"=73, "Sensor Velocity"=74, "Current"=75, "Brake is Enabled"=76, "Encoder Position"=77, "Encoder Velocity"=78, "Encoder Index Rise Events"=79, "Encoder A Pin State"=80, "Encoder B Pin State"=81, "Encoder Index Pin State"=82, "Analog In with Overflow"=83, "Analog In Velocity"=84, "Temperature"=85, "Battery Voltage"=86, "Reset Count"=87, "Reset Flags"=88, "Firmware Version"=89, "Settings Changed"=90, "Quad Filter Enable"=91, "Ignore Disable Broadcast"=92, "I Accumulator"=93, "Status 1 Frame Rate Ms"=94, "Status 2 Frame Rate Ms"=95, "Status 3 Frame Rate Ms"=96, "Status 4 Frame Rate Ms"=97, "Status 6 Frame Rate Ms"=98, "Status 7 Frame Rate Ms"=99, "Enable Index Pin Clear Position"=100, "Peak Positive Output"=104, "Nominal Positive Output"=105, "Peak Negative Output"=106, "Nominal Negative Output"=107, "Quad Index Pin Polarity"=108, "Status 8 Frame Rate Ms"=109, "Allow Position Overflow"=110, "Slot 0 - Allowable Closed-Loop Error"=111, "Number Potentiometer Turns"=112, "Encoder Codes Per Rev"=113, "Pulse Width Decoded Position"=114, "Analog Position"=115, "Voltage Compensation Rate (V/s)"=116, "Slot 1 - Allowable Closed-Loop Error"=117, "Motion Profile Has Underrun Err"=119, "Reserved 120"=120, "Legacy Control Mode"=121, "Motion Magic Acceleration"=122, "Motion Magic Cruise Velocity"=123, "Status 10 Frame Rate"=124, "Current Limit Threshold"=125, "CustomParam0"=137, "CustomParam1"=138, "PersStorageSaving"=139, "ClearPositionOnLimitF"=144, "ClearPositionOnLimitR"=145, "NominalBatteryVoltage"=146, "SampleVelocityPeriod"=147, "SampleVelocityWindow"=148] ("Parameter")
          n205 = Unbundle By Name(w524) -> ("CAN.Device Number"=w521:u8)
          n206 = Unbundle By Name(w522) -> ("CAN.Device Number"=w523:u8)
          n207 = call <vilib>:"WPI_CANTalonSRX_SetParameter.vi"("Value"=0.0, "Parameter"=w527, "Device ID (0)"=w521) -> ()  [unwired: 7 in, 2 out]
          n208 = call <vilib>:"WPI_CANTalonSRX_SetParameter.vi"("Value"=0.0, "Parameter"=w526, "Device ID (0)"=w523) -> ()  [unwired: 7 in, 2 out]
        }
      }
    }
    frame "Forward" {
      n209 = call-poly <vilib>:"WPI_RobotDriveArcadeDrive.vi"("error in (no error)"=w533, "Y axis value"=0.55, "RobotDriveDevRef"=w534) -> ("error out"=w529:errorcluster, "RobotDriveDevRef"=w531:T9)  [unwired: 6 in, 1 out]
      n210 = call <vilib>:"WPI_RobotDriveDelayAndUpdateSafety.vi"("error in (no error)"=w529, "Delay (s)"=2.8, "RobotDriveDevRef"=w531) -> ()  [unwired: 7 in, 2 out]
    }
    frame "GEAR DROP" {
      n211 = call-poly <vilib>:"WPI_RobotDriveArcadeDrive.vi"("error in (no error)"=w558, "Y axis value"=0.45, "RobotDriveDevRef"=w559) -> ("error out"=w555:errorcluster, "RobotDriveDevRef"=w556:T9)  [unwired: 6 in, 1 out]
      n212 = call <vilib>:"WPI_RobotDriveDelayAndUpdateSafety.vi"("error in (no error)"=w555, "Delay (s)"=2.4, "RobotDriveDevRef"=w556) -> ("error out"=w553:errorcluster, "RobotDriveDevRef 2"=w552:T9)  [unwired: 7 in]
      n213 = call-poly <vilib>:"WPI_RobotDriveArcadeDrive.vi"("error in (no error)"=w553, "Y axis value"=0.0, "RobotDriveDevRef"=w552) -> ("error out"=w549:errorcluster, "RobotDriveDevRef"=w550:T9)  [unwired: 6 in, 1 out]
      n214 = call <vilib>:"WPI_RobotDriveDelayAndUpdateSafety.vi"("error in (no error)"=w549, "Delay (s)"=0.5, "RobotDriveDevRef"=w550) -> ("error out"=w542:errorcluster, "RobotDriveDevRef 2"=w541:T9)  [unwired: 7 in]
      n215 = while {
        tunnel: w542 -> [w571]
        tunnel: [w568] -> w540
        tunnel: w539 -> [w567]
        tunnel: [w566] -> w538
        stop <- w569 stop-if-true
        n216 = global read "Robot Global Data.vi" "LOWER LIMIT"() -> (w569:bool)
        n217 = call <vilib>:"WPI_MotorControlSetOutput.vi"("error in (no error)"=w571, "Output"=-0.6 ("f"), "MotorControlDevRef"=w567) -> ("error out"=w568:errorcluster, "MotorControlDevRef"=w566:T4)  [unwired: 6 in, 1 out]
      }
      n218 = call-poly <vilib>:"WPI_RobotDriveArcadeDrive.vi"("error in (no error)"=w540, "Y axis value"=-0.4, "RobotDriveDevRef"=w541) -> ("error out"=w546:errorcluster, "RobotDriveDevRef"=w545:T9)  [unwired: 6 in, 1 out]
      n219 = call <vilib>:"WPI_RobotDriveDelayAndUpdateSafety.vi"("error in (no error)"=w546, "Delay (s)"=1.5, "RobotDriveDevRef"=w545) -> ("error out"=w537:errorcluster)  [unwired: 7 in, 1 out]
      n220 = while {
        tunnel: w538 -> [w564]
        tunnel: w537 -> [w562]
        tunnel: [w561] -> w536
        tunnel: [w560] -> w535
        stop <- w565 stop-if-true
        n221 = call <vilib>:"WPI_MotorControlSetOutput.vi"("error in (no error)"=w562, "Output"=0.6, "MotorControlDevRef"=w564) -> ("error out"=w560:errorcluster, "MotorControlDevRef"=w561:T4)  [unwired: 6 in, 1 out]
        n222 = global read "Robot Global Data.vi" "UPPER LIMIT"() -> (w565:bool)
      }
      n223 = call <vilib>:"WPI_MotorControlSetOutput.vi"("error in (no error)"=w535, "Output"=0.0, "MotorControlDevRef"=w536) -> ()  [unwired: 6 in, 3 out]
    }
  }
